vi "VPIExtraction.vi"() -> ()   [LabVIEW 2022 SP3]
uses:
  -planewaveSubs/VPIParams.ctl
  ViewData/-ReadEye/Header.ctl
  <vilib>/Utility/miscctls.llb/LVPointDoubleTypeDef.ctl
  <vilib>/Utility/error.llb/DialogType.ctl
  <vilib>/vision/Avi.llb/IMAQ AVI2 Codec Path.ctl
  ViewData/-ReadEye/TypeDefs/TypeofMean.ctl
  <vilib>/Analysis/baseanly.llb/Mean (DBL).vi
  <vilib>/Analysis/2dsp.llb/Decimate (single shot, DBL).vi
  <vilib>/Analysis/baseanly.llb/Normalize Matrix.vi
  <vilib>/Utility/file.llb/Write Delimited Spreadsheet (DBL).vi
  <vilib>/Utility/file.llb/Write Delimited Spreadsheet (string).vi
  <vilib>/Analysis/NI_AALBase.lvlib
  <vilib>/Analysis/NI_AALPro.lvlib
panel:
  in  "y scale Circ":sgl=1.0
  in  "Circle Mask":bool
  in  "RMS":bool
  in  "B1 Set":bool
  out "Header In":T1={"header info"={"Header"="", "Head length"=0}, "A/D info"={"# rf points per line"=0, "# lines per scan"=0, "sample rate MHz"=0, "# A/D bits"=0, "# bytes per A/D"=0, "TGC Flag"=0, "A/D Type"=""}, "Tranducer Info"={"bandwidth"=0.0, "center freq"=0.0, "start freq"=0.0, "ID"=0}, "Scan Info"={"delay"=0.0, "pivot distance"=0.0, "sector scan angle"=0.0, "operator"="", "Scan Mode"="", "location"=""}, "Time/Date Info"={"date"="", "time"=""}, "RF Info"={"RF file name"="", "RF file att"="", "RF cal file name"="", "RF cal file att"=""}, "Patient Info"={"ID"="", "extended ID"="", "age"=0, "sex"="", "previously\nscanned"="", "PSA"=0.0, "LOS"=1, "Ethnicty 2"=3, "Race"=3}, "Tissue Type"={"organ"=0, "disease type"=0, "disease location"=0, "IQ_pts"=0, "RcvBuffer"=0, "RcvFrame"=0, "IQBuff"=0, "IQFrame"=0, "IQPage"=0}, "Votage scaling"={"Digitizer (dB)"=0.0, "Gain (dB)"=0.0, "Atten (dB)"=0.0}, "Comment"="", "Misc Info"={"avg num"=0, "c speed"=0, "Div By or SF zones"=0, "XMIT CHS"=0, "RCV CHS"=0, "Xmit angle"=0.0}, "Therapy Parameters"={"Theraputic Freq (MHz)"=0.0, "Time on (s)"=0.0, "Therapy amplitude (mV)"=0.0, "Lines Before"=0, "Lines After"=0}, "Scan Settings"={"Energy (uJ or V)"=0, "Damp (Ohm) or Fc"=0, "HP Filt (KHz)"=0, "LP Filt (MHz)"=0, "Gain (db)"=0, "prf (kHz)"=0.0, "Distance between\nscan lines (um)"=0, "Distance between\nscan planes (um)"=0, "Scan line gap (um)"=0.0, "Scan plane gap (um)"=0.0}, "Compression Parameters"={"F1 (MHz)"=0.0, "F2 (MHz)"=0.0, "% taper"=0.0, "duration"=0.0}, "Patient Info Xtra"={"First Name"="", "Last Name"="", "Notes"=""}, "ROI Box"=[0, 0, 0, 0]} {"Compression Parameters"."% taper" min=50 max=1000 format="%.2f"; "Compression Parameters"."F2 (MHz)" format="%.3f"; "Compression Parameters"."F1 (MHz)" format="%.3f"; "Scan Settings"."prf (kHz)" format="%.2f"; "Therapy Parameters"."Therapy amplitude (mV)" min=50 max=1000 format="%.2f"; "Therapy Parameters"."Time on (s)" format="%.3f"; "Therapy Parameters"."Theraputic Freq (MHz)" format="%.3f"; "Patient Info"."Race" items=["Am Ind or Alaska", "Asian", "Hawaiian, Pac Isl", "Black or Afr Amer", "White", "more than one race", "unknown"]; "Patient Info"."Ethnicty 2" items=["Hispanic", "Non-Hispanic", "unknown"]; "Patient Info"."LOS" items=["1", "2", "3", "4", "5"]; "Patient Info"."PSA" format="%.1f"; "Scan Info"."delay" format="%.2f"; "Scan Info"."pivot distance" format="%.2f"; "Scan Info"."sector scan angle" format="%.2f"; "Tranducer Info"."bandwidth" format="%.2f"; "Tranducer Info"."center freq" format="%.2f"; "Tranducer Info"."start freq" format="%.2f"}
  in  "EKG Trace":path
  in  "No Mask?":bool=TRUE
  in  "Range Control":T2={"Vel Range"={1.4018691588785046, 50.0}, "PFlow Range"={22.429906542056074, 90.28037383177569}, "IQ Range"={28.037383177570092, 102.05607476635514}, "ShortLag"={33.08411214953271, 88.59813084112149}, "Mean Pow"={0.0, 41.12149532710281}, "powT"={0.0, 41.12149532710281}, "varT"={0.0, 41.12149532710281}} {"varT" scale=0.0..100.0; "powT" scale=0.0..700.0; "Mean Pow" scale=0.0..100.0; "ShortLag" scale=0.0..120.0; "IQ Range" scale=-25.0..120.0; "PFlow Range" scale=0.0..120.0; "Vel Range" scale=-1.0..150.0}
  in  "Main Tab":enum32{"Page 1", "Page 2", "Page 4"}(tab)=enum."Page 2"
  out "output cluster":T3
  out "powT":sgl[][](graph)
  out "VarT":sgl[][](graph)
  out "IQData (thresholdC=powerCMap)":sgl[][](graph)
  out "Mean varS":sgl[][](graph)
  out "powerFlow line":sgl[](graph)
  out "Short lag vs slow time VarS":sgl[](graph)
  out "Short lag variance VarS":sgl[][](graph)
  out "powerFlow (threshold = avg Var)":sgl[][](graph)
  out "Mean Pow":sgl[][](graph)
  out "Mean PowT":sgl[][](graph)
  out "Histogram Graph":T4(graph)
  in  "Max V":i32(slide)=24 scale=0.0..60.0
  in  "Save VPI JPGs":bool
  in  "Save Vels":bool
  out "Vel Y (cm/s) Main":sgl[][](graph)
  out "Velocity  vs time (cm/s)":dbl[][](graph)
  in  "AVG":i32=1 min=1
  in  "Operation":u16(ring) items=["Median", "Mean"]
  out "Vector Image":T5(plugin-control)
  out "SG":picture
  out "SG File":string
  out "Current  VPI":string
  in  "Card Cycles":i32=1
  out "CD Image":T5(plugin-control)
  in  "Location note":string
  in  "Skip":dbl=4.0
  in  "Skip overide?":bool
  out "Skip File":dbl
  in  "Tab Display":T6(tab)=enum."V at Marker"
  out "Vel Y (cm/s) Ref":sgl[][](graph)
  out "Vel mag (cm/s)":sgl[][](graph)
  out "Vel X (cm/s) Ref":sgl[][](graph)
  out "phase (cm/s)":sgl[][](graph)
  out "Raw Filtered":sgl[][](graph)
  in  "Frame":i32
  out "Velocity spread":cluster{"Y":dbl[], "Y":dbl[]}[](graph)
  out "Vel Sum (cm/s)":T7 {"Plane" min=0 step=1; "Curs Y" min=0 step=1; "Curs X" min=0 step=1}
  out "VelT":dbl[](graph)
  in  "length":i32=10
  in  "VPI Fix":cluster{"Offset":T8, "Scale":T8}={"Offset"={"X"=38.0, "Y"=10.0}, "Scale"={"X"=0.64, "Y"=0.82}}
  in  "CD Fix":cluster{"Offset":T8, "Scale":T8}={"Offset"={"X"=21.0, "Y"=19.0}, "Scale"={"X"=0.7, "Y"=0.673}}
  in  "SG Fix":cluster{"Start":dbl, "scale":dbl}={"Start"=55.0, "scale"=0.213}
  out "Velocity cut x-y plane (cm/s)":dbl[][](graph)
  out "Velocity cut  mean\nall time(cm/s)":dbl[][](graph)
  out "Flow Phase vs time":dbl[](graph)
  out "V mean running":dbl[][](array[numeric])
  out "V mean Var":dbl[][](array[numeric])
  out "Average vorticity vs time rot/s":dbl[][](graph)
  out "Energy loss vs time in window":dbl[](graph)
  in  "center zero":i32
  out "error%":dbl
  in  "rev/s":dbl=6.0
  out "mean vorticity":dbl format="%0.2f"
  out "Vorticity slow time":dbl[](graph)
  out "vorticy pixel\nmean across time":dbl format="%0.2f"
  in  "AVG #":i32=1 min=1
  in  "Vort Mean/Median":u16(ring) items=["Median", "Mean"]
  in  "vort frame  average":i32=3
  in  "step vort":i32=5
  in  "mean vort":bool
  in  "Save Vortex":bool
  out "KE vs time":dbl[](graph)
  in  "vort add char":string
  in  "downsamp factor":i32=10
  out "EKG":picture
  out "Peak Tracker":dbl[][](graph)
  in  "2D threshold":sgl=20.0
  in  "Ref Frame 2D CC":i32
  in  "#y rf":i32=80
  in  "#x lines":i32=100
  out "Simple Motion Tracker":dbl[](graph)
  out "Raw data (motion track marks)":sgl[][](graph)
  out "2D Correlation":dbl[][](graph)
  out "BPM":i32
  in  "True Center Freq":dbl=15.5
  in  "Save Images":bool
  in  "ImageSavePath":path=path "E:/Papers/IEEE/2109 VPI LV/FigsData"
  in  "VPI Case":i32 min=0
  out "Current":i32
  out "Total":i32
  out "Direction Map":picture
  in  "Direction cColor":picture
  in  "vort min val":dbl(slide) scale=0.0..1000.0
  out "z grid":cdb[][](array[numeric])
  in  "Values":T9
  in  "Plane":i32 min=0 step=1
  in  "stop":bool
  in  "Use Selected Files":bool
  in  "Listbox":i32[](listbox)
  in  "directory path of data and header file":path
  in  "search pattern":string="*VPI.raw"
  # "17.857 ref"
  # "Color based on net axial up or down"
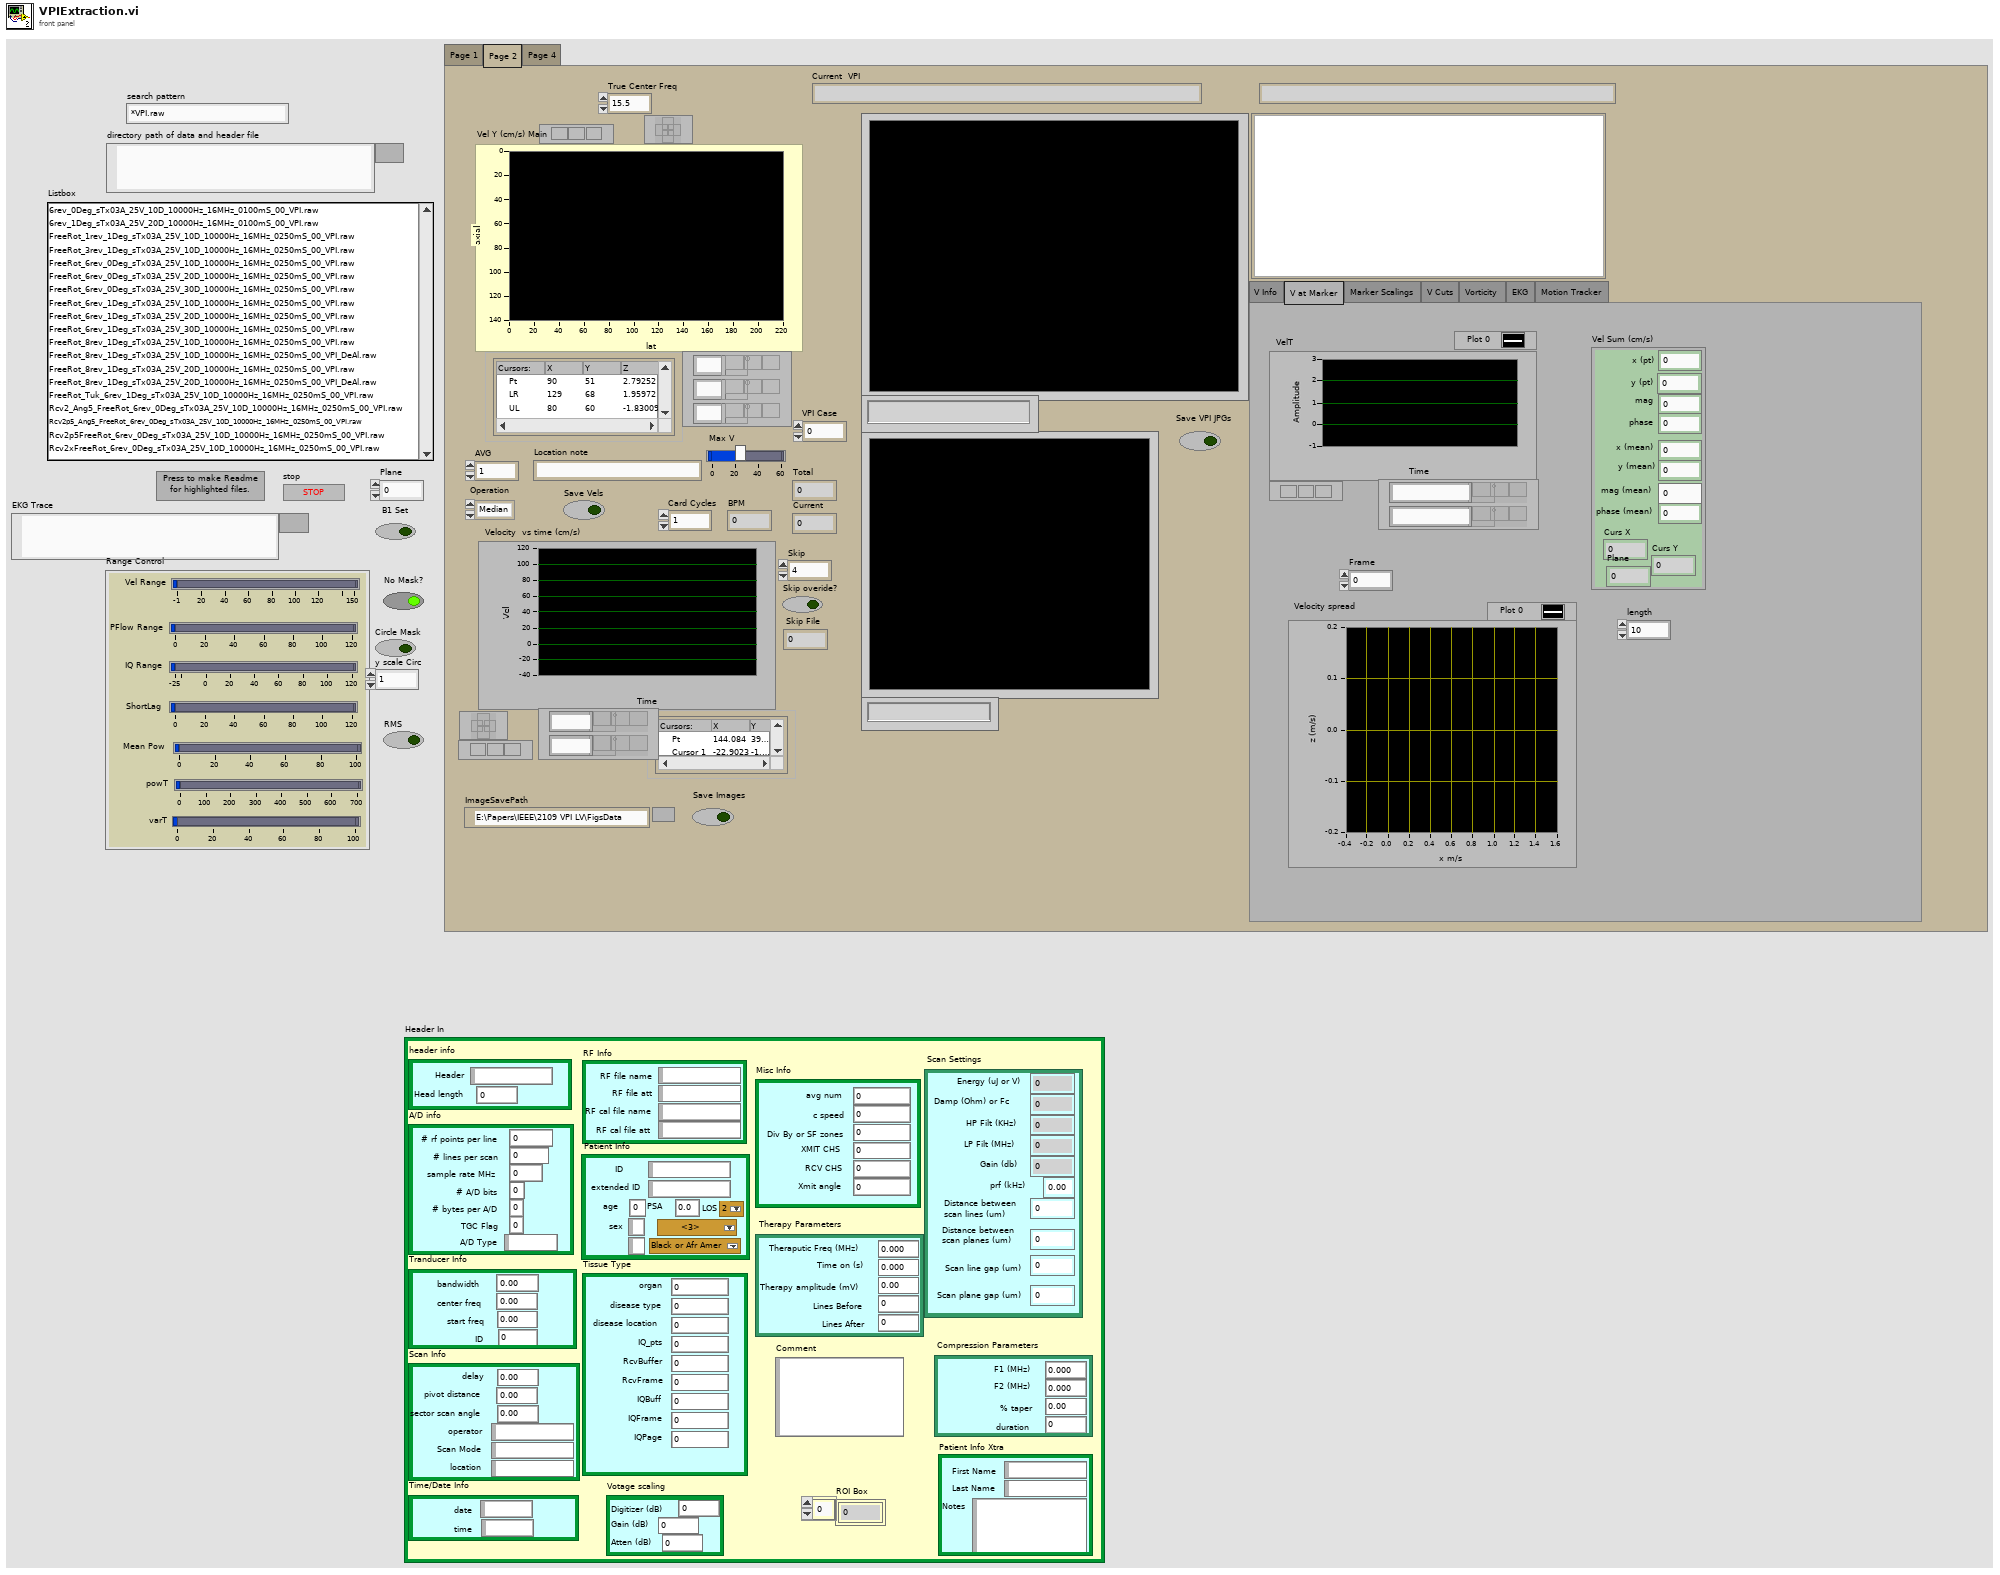
[diagram p1: front panel]
types:
  T1 = typedef "Header.ctl" = cluster{"header info":cluster{"Header":string, "Head length":i16}, "A/D info":cluster{"# rf points per line":u16, "# lines per scan":u16, "sample rate MHz":u16, "# A/D bits":i16, "# bytes per A/D":u16, "TGC Flag":u16, "A/D Type":string}, "Tranducer Info":cluster{"bandwidth":sgl, "center freq":sgl, "start freq":sgl, "ID":i32}, "Scan Info":cluster{"delay":sgl, "pivot distance":sgl, "sector scan angle":sgl, "operator":string, "Scan Mode":string, "location":string}, "Time/Date Info":cluster{"date":string, "time":string}, "RF Info":cluster{"RF file name":string, "RF file att":string, "RF cal file name":string, "RF cal file att":string}, "Patient Info":cluster{"ID":string, "extended ID":string, "age":u16, "sex":string, "previously\nscanned":string, "PSA":sgl, "LOS":u8, "Ethnicty 2":u8, "Race":u8}, "Tissue Type":cluster{"organ":i16, "disease type":i16, "disease location":i16, "IQ_pts":u16, "RcvBuffer":u8, "RcvFrame":u16, "IQBuff":u8, "IQFrame":u16, "IQPage":u8}, "Votage scaling":cluster{"Digitizer (dB)":sgl, "Gain (dB)":sgl, "Atten (dB)":sgl}, "Comment":string, "Misc Info":cluster{"avg num":u16, "c speed":i16, "Div By or SF zones":i16, "XMIT CHS":u8, "RCV CHS":u8, "Xmit angle":sgl}, "Therapy Parameters":cluster{"Theraputic Freq (MHz)":sgl, "Time on (s)":sgl, "Therapy amplitude (mV)":sgl, "Lines Before":u16, "Lines After":u16}, "Scan Settings":cluster{"Energy (uJ or V)":u8, "Damp (Ohm) or Fc":u8, "HP Filt (KHz)":u8, "LP Filt (MHz)":u8, "Gain (db)":u8, "prf (kHz)":sgl, "Distance between\nscan lines (um)":u16, "Distance between\nscan planes (um)":u16, "Scan line gap (um)":sgl, "Scan plane gap (um)":sgl}, "Compression Parameters":cluster{"F1 (MHz)":sgl, "F2 (MHz)":sgl, "% taper":sgl, "duration":sgl}, "Patient Info Xtra":cluster{"First Name":string, "Last Name":string, "Notes":string}, "ROI Box":u16[]}
  T2 = cluster{"Vel Range":cluster{dbl, dbl}, "PFlow Range":cluster{dbl, dbl}, "IQ Range":cluster{dbl, dbl}, "ShortLag":cluster{dbl, dbl}, "Mean Pow":cluster{dbl, dbl}, "powT":cluster{dbl, dbl}, "varT":cluster{dbl, dbl}}
  T3 = cluster{"Vel Max":sgl, "Vel Min":sgl, "PF Max":sgl, "PF Min":sgl, "IQ Max":sgl, "IQ Min":sgl, "ShortLag Max":sgl, "ShortLag Min":sgl, "MeanPow Max":sgl, "MeanPow Min":sgl, "powT max":sgl, "powT min":sgl, "varT max":sgl, "varT min":sgl}
  T4 = cluster{"X Values":dbl[], "Histogram: h(x)":i32[]}
  T5 = typedef "IMAQ Image.ctl" = refnum<image>
  T6 = enum32{"V Info", "V at Marker", "Marker Scalings", "V Cuts", "Vorticity", "EKG", "Motion Tracker"}
  T7 = cluster{"x (pt)":sgl, "y (pt)":sgl, "mag":sgl, "phase":sgl, "x (mean)":sgl, "y (mean)":sgl, "mag (mean)":sgl, "phase (mean)":sgl, "Curs X":sgl, "Curs Y":sgl, "Plane":sgl}
  T8 = typedef "LVPointDoubleTypeDef.ctl" = cluster{"X":dbl, "Y":dbl}
  T9 = typedef "VPIParams.ctl" = cluster{"xdim":dbl, "ydim":dbl, "zdim":dbl, "skip":dbl, "ensembleC":dbl, "ensembleVar\n":dbl, "#tx":dbl, "#Rx":dbl, "deltaX":dbl, "deltaY":dbl, "x start":dbl, "ystart":dbl}
  T10 = enum16{"big-endian, network order", "native, host order", "little-endian"}
  T11 = typedef "DialogType.ctl" = u16
  T12 = typedef "IMAQ AVI2 Codec Path.ctl" = u32
  T13 = typedef "IMAQ AVI2 Refnum.ctl" = refnum<k20>
  T14 = typedef "Image Type" = u32
  T15 = cluster{"AVI Refnum (duplicate)":T13, "New Image":T5, "appended path":path, sgl[][][], csg[][][], sgl[][][], "Values":T9, sgl[][][], "mean pow ":sgl[][], "mean var":sgl[][], "AVI Refnum (duplicate)":T13, "New Image":T5, "Number of Frames":u32, "Number of Frames":u32, sgl[][][], sgl[][][], sgl[][][], sgl[][][], "Header In":T1, "result string":string, sgl[][][]}
  T16 = typedef "TypeofMean.ctl" = enum16{"Mean from lines", "Mean just lines", "Poly Mean", "No mean", "Filter"}
  T17 = cluster{"abs(IQ)":sgl[][], "abs(IQ) SVD":sgl[][], "Vector out":csg[][], "pow":sgl[][], "vars short lag":sgl[][], "powT":sgl[][], "varT":sgl[][]}
  T18 = cluster{dbl, dbl, dbl, dbl, sgl, sgl, sgl, sgl, "Cursor X":dbl, "Cursor Y":dbl, "Plane":i32}
  T19 = typedef "NI_Matrix.lvlib/RealMatrix.ctl" = dbl[][]
  T20 = typedef "imagedata.ctl" = cluster{"image type":i32, "image depth":i32, "image":u8[], "mask":u8[], "colors":u32[], "Rectangle":cluster{"left":i16, "top":i16, "right":i16, "bottom":i16}}
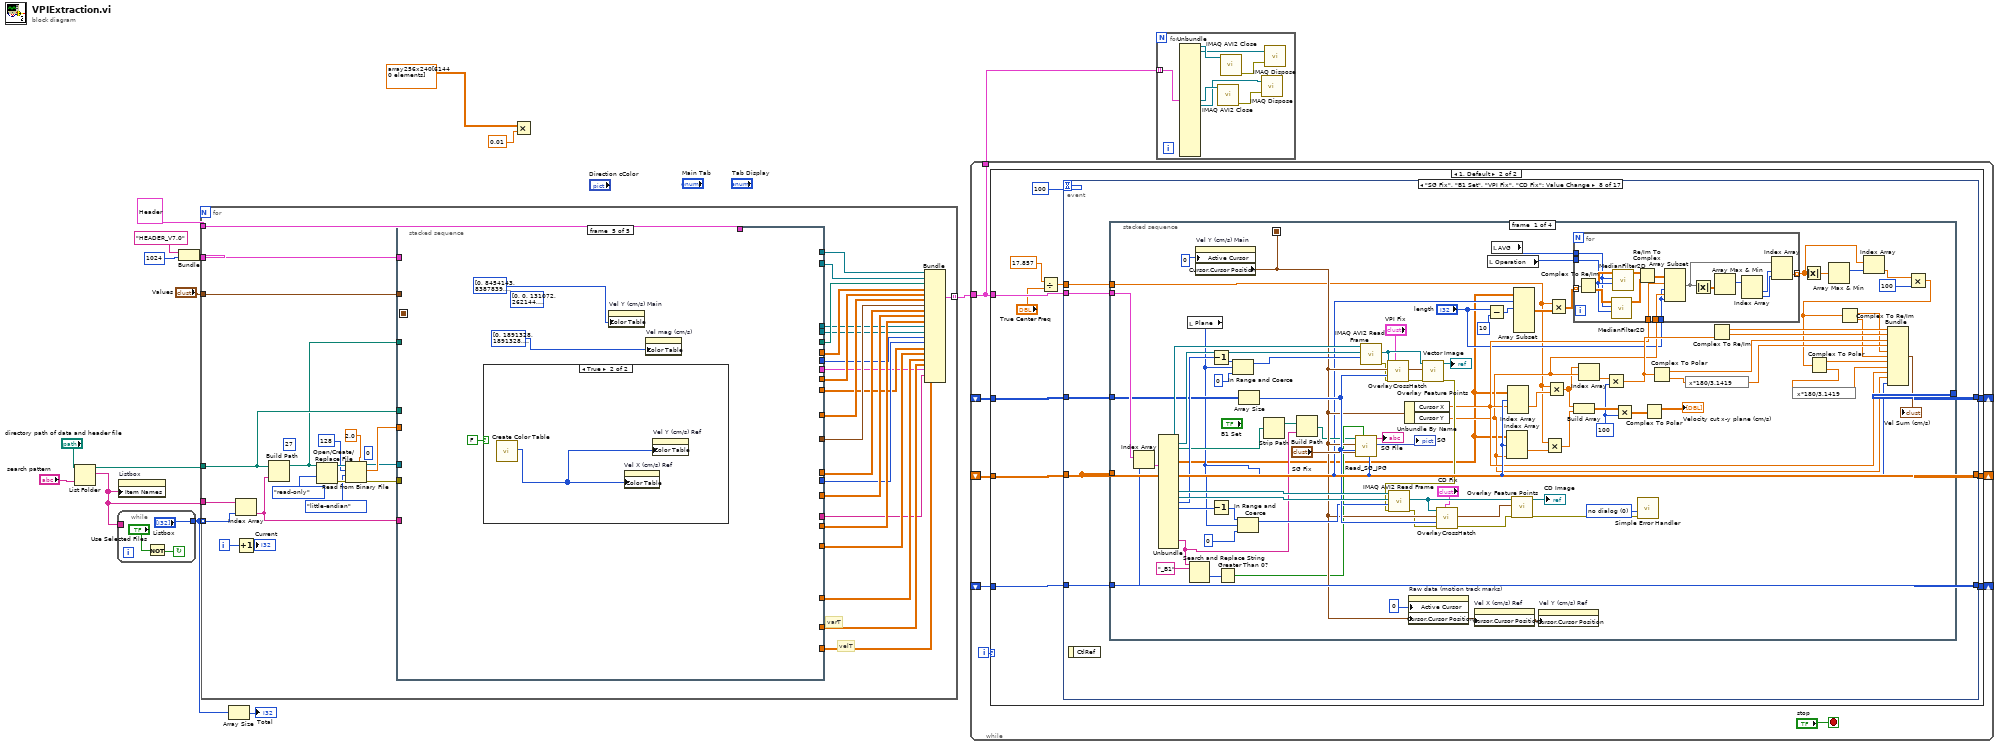
[diagram p0: block diagram]
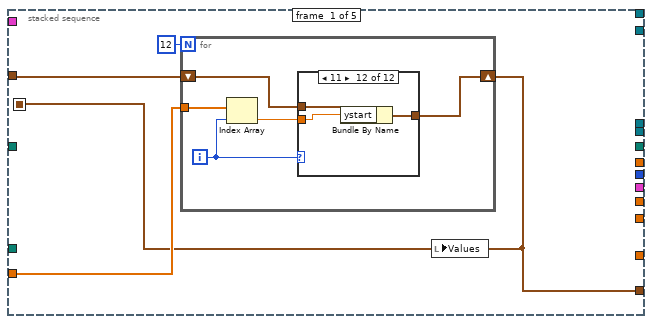
[diagram p2: hidden frame]
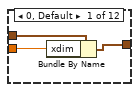
[diagram p3: hidden frame]
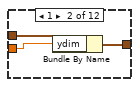
[diagram p4: hidden frame]
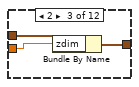
[diagram p5: hidden frame]
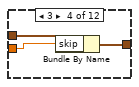
[diagram p6: hidden frame]
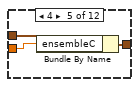
[diagram p7: hidden frame]
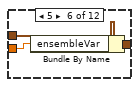
[diagram p8: hidden frame]
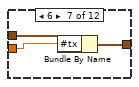
[diagram p9: hidden frame]
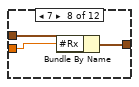
[diagram p10: hidden frame]
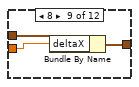
[diagram p11: hidden frame]
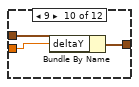
[diagram p12: hidden frame]
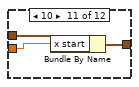
[diagram p13: hidden frame]
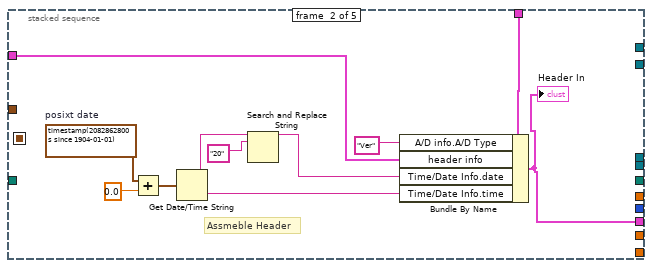
[diagram p14: hidden frame]
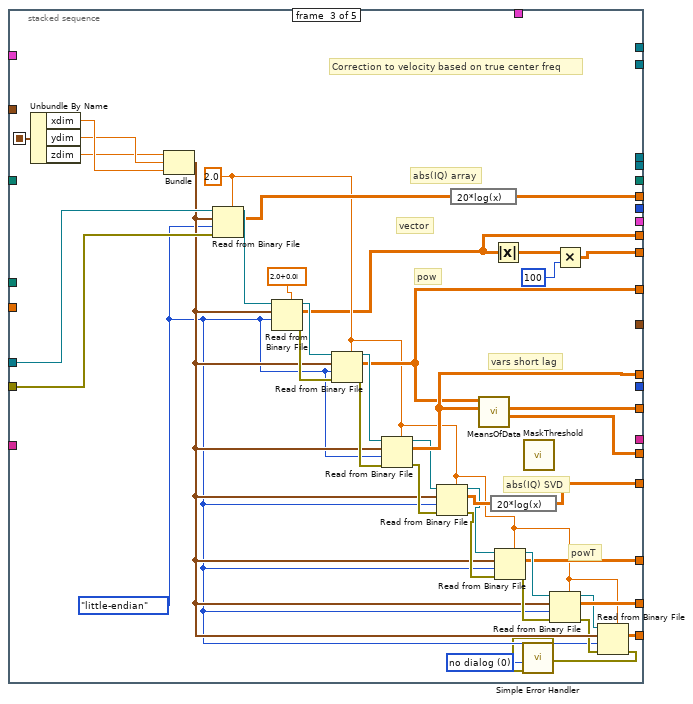
[diagram p15: hidden frame]
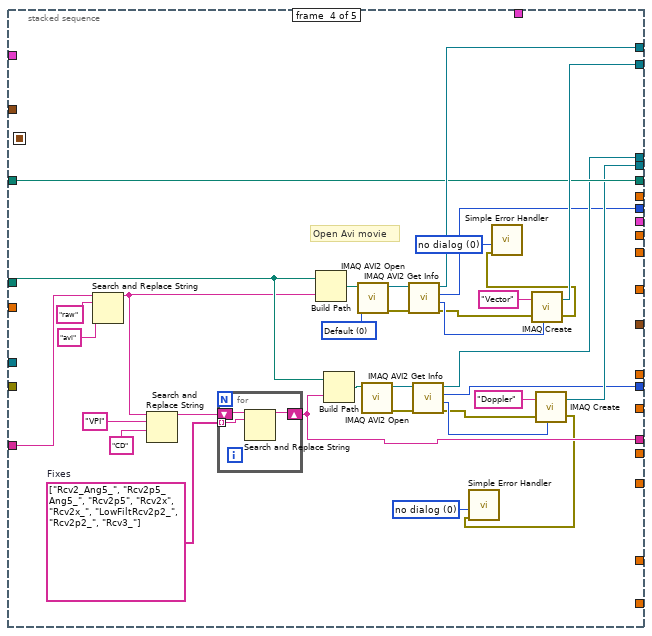
[diagram p16: hidden frame]
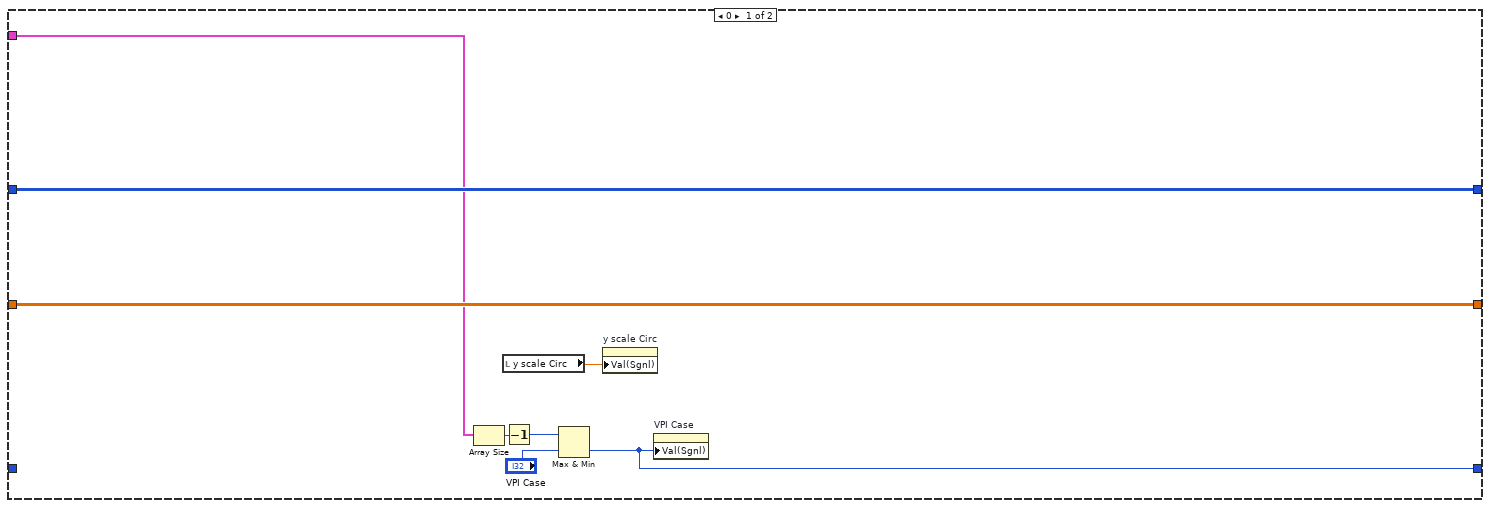
[diagram p18: hidden frame]
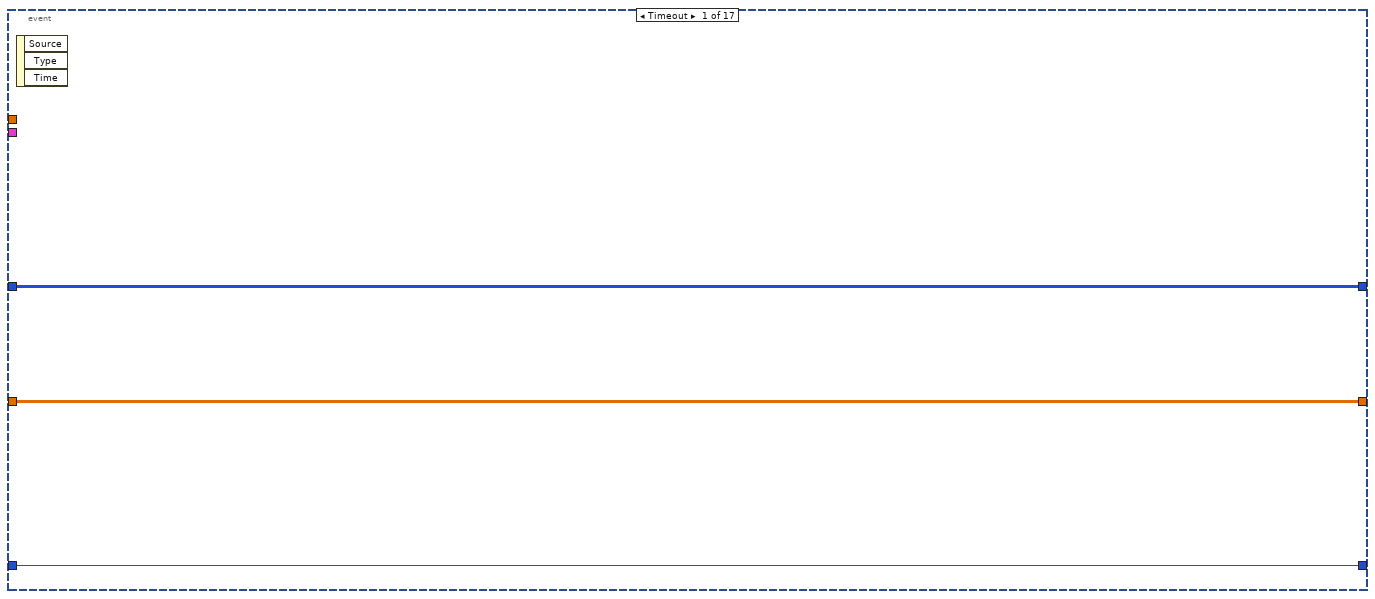
[diagram p19: hidden frame]
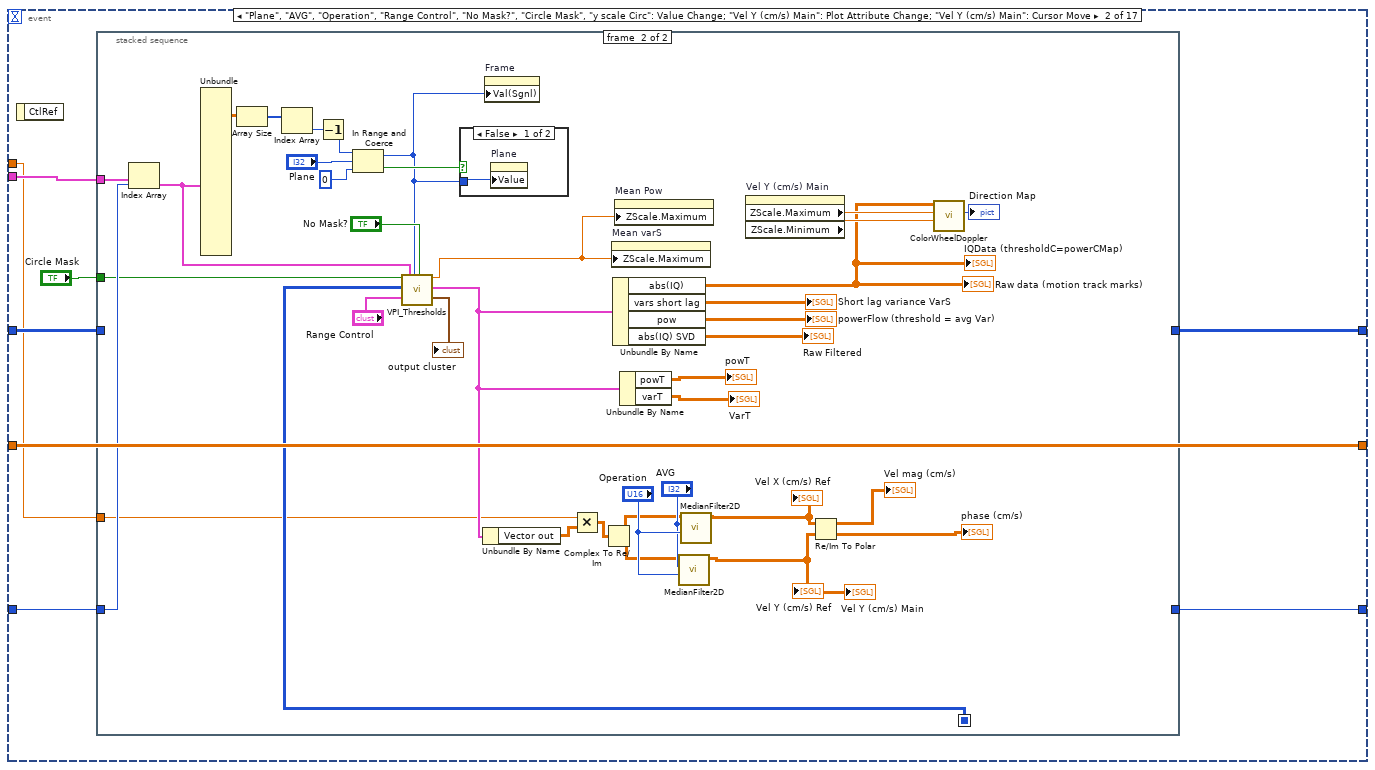
[diagram p20: hidden frame]
diagram:
  n1 = List Folder(path="directory path of data and header file", pattern="search pattern") -> (path out=w12:path, filenames=w11:string[])  [unwired: 1 in, 3 out]
  n2 = while {
    tunnel: ["Listbox"] -> w4
    tunnel: w11 -> [_]
    stop <- w18 continue-if-true
    n3 = Not(x="Use Selected Files") -> (.not. x?=w18:bool)
  }
  n4 = property on="Listbox" class="LstBox (strict)"("Item Names"=w11) -> ()  [unwired: 2 in, 2 out]
  n5 = Bundle("HEADER_V7.0", 1024) -> (w7:cluster{string, i32})  [unwired: 1 in]
  n6 = for {
    tunnel: w4 -> [w59] mode=indexing
    tunnel: w11 -> [w58]
    tunnel: w12 -> [w44]
    tunnel: T1 {"header info"={"Header"="", "Head length"=0}, "A/D info"={"# rf points per line"=0, "# lines per scan"=0, "sample rate MHz"=0, "# A/D bits"=0, "# bytes per A/D"=0, "TGC Flag"=0, "A/D Type"=""}, "Tranducer Info"={"bandwidth"=0.0, "center freq"=0.0, "start freq"=0.0, "ID"=0}, "Scan Info"={"delay"=0.0, "pivot distance"=0.0, "sector scan angle"=0.0, "operator"="", "Scan Mode"="", "location"=""}, "Time/Date Info"={"date"="", "time"=""}, "RF Info"={"RF file name"="", "RF file att"="", "RF cal file name"="", "RF cal file att"=""}, "Patient Info"={"ID"="", "extended ID"="", "age"=0, "sex"="", "previously\nscanned"="", "PSA"=0.0, "LOS"=1, "Ethnicty 2"=3, "Race"=3}, "Tissue Type"={"organ"=0, "disease type"=0, "disease location"=0, "IQ_pts"=0, "RcvBuffer"=0, "RcvFrame"=0, "IQBuff"=0, "IQFrame"=0, "IQPage"=0}, "Votage scaling"={"Digitizer (dB)"=0.0, "Gain (dB)"=0.0, "Atten (dB)"=0.0}, "Comment"="", "Misc Info"={"avg num"=0, "c speed"=0, "Div By or SF zones"=0, "XMIT CHS"=0, "RCV CHS"=0, "Xmit angle"=0.0}, "Therapy Parameters"={"Theraputic Freq (MHz)"=0.0, "Time on (s)"=0.0, "Therapy amplitude (mV)"=0.0, "Lines Before"=0, "Lines After"=0}, "Scan Settings"={"Energy (uJ or V)"=0, "Damp (Ohm) or Fc"=0, "HP Filt (KHz)"=0, "LP Filt (MHz)"=0, "Gain (db)"=0, "prf (kHz)"=0.0, "Distance between\nscan lines (um)"=0, "Distance between\nscan planes (um)"=0, "Scan line gap (um)"=0.0, "Scan plane gap (um)"=0.0}, "Compression Parameters"={"F1 (MHz)"=0.0, "F2 (MHz)"=0.0, "% taper"=0.0, "duration"=0.0}, "Patient Info Xtra"={"First Name"="", "Last Name"="", "Notes"=""}, "ROI Box"=[0, 0, 0, 0]} ("Header In") -> [w57]
    tunnel: w7 -> [w56]
    tunnel: "Values" -> [w49]
    tunnel: [w32] -> w15 mode=indexing
    i -> [w27]
    (unwired) u32 27 ("Column/Row to Sort By")
    (unwired) i64 0 ("offset (in bytes)")
    # "velT"
    # "varT"
    n7 = Index Array(array=w58, index=w59) -> (element=w45:string)
    n8 = Increment(x=w27) -> (x+1=→"Current":i32)
    n9 = Build Path(base path=w44, name or relative path=w45) -> (appended path=w43:path)
    n10 = Open/Create/Replace File(file path (use dialog)=w43, access (0:read/write)=enum16{"read/write", "read-only", "write-only"}."read-only") -> (refnum out=w54:refnum<file>, error out=w53:errorcluster)  [unwired: 4 in, 1 out]
    n11 = Read from Binary File(5:sgl 2.0 ("double"), 8:w53, 9:T10."little-endian" ("byte order (0:big-endian, network order)"), 10:128 ("count (1)"), 11:w54) -> (0:w47:errorcluster, 2:w50:sgl[], 3:w48:refnum<file>)  [unwired: 1 in, 1 out]
    n12 = stacked-sequence {
      seq-local: [w60 _ _ _ _] -> [_ _ w153 _ _]
      tunnel: w57 -> [_ w115 _ _ _]
      tunnel: w56 -> [_ w108 _ _ _]
      tunnel: w50 -> [w63 _ _ _ _]
      tunnel: w49 -> [w61 _ _ _ _]
      tunnel: w48 -> [_ _ w155 _ _]
      tunnel: w47 -> [_ _ w154 _ _]
      tunnel: [_ _ w143 _ _] -> w39
      tunnel: [_ _ w141 _ _] -> w37
      tunnel: [_ _ w116 _ _] -> w38
      tunnel: [_ _ w142 _ _] -> w35
      tunnel: [w60 _ _ _ _] -> w36
      tunnel: [_ _ w139 _ _] -> w33
      tunnel: [_ _ w140 _ _] -> w34
      tunnel: w45 -> [_ _ _ w165 _]
      tunnel: w44 -> [_ _ _ w172 _]
      tunnel: [_ _ _ w182 _] -> w41
      tunnel: [_ _ _ w181 _] -> w42
      tunnel: [_ _ _ w180 _] -> w40
      tunnel: w43 -> [_ _ _ w180 _]
      tunnel: [_ _ _ w170 _] -> w30
      tunnel: [_ _ _ w169 _] -> w31
      tunnel: [_ _ _ w168 _] -> w29
      tunnel: [_ _ _ w167 _] -> w28
      tunnel: [_ _ w136 _ _] -> w25
      tunnel: [_ _ w132 _ _] -> w24
      tunnel: [_ _ w127 _ _] -> w23
      tunnel: [_ _ w126 _ _] -> w22
      tunnel: [_ w105 _ _ _] -> w21
      tunnel: [_ _ _ w162 _] -> w20
      tunnel: [_ _ w119 _ _] -> w19
      frame #0 {
        n13 = for {
          N: 12 -> [_]
          tunnel: w63 -> [w68]
          shift-right: [w65] -> w60
          shift-left: w61 -> [w64]
          i -> [w66]
          n14 = Index Array(array=w68, index=w66) -> (element=w67:sgl)
          n15 = case shown="11" w66 {
            tunnel: w67 -> [w71 w74 w77 w80 w83 w86 w89 w92 w95 w98 w101 w104]
            tunnel: [w70 w73 w76 w79 w82 w85 w88 w91 w94 w97 w100 w103] -> w65
            tunnel: w64 -> [w69 w72 w75 w78 w81 w84 w87 w90 w93 w96 w99 w102]
            frame 0, Default {
              n16 = Bundle By Name(cluster=w69, "xdim"=w71) -> (w70:T9)
            }
            frame 1 {
              n17 = Bundle By Name(cluster=w72, "ydim"=w74) -> (w73:T9)
            }
            frame 2 {
              n18 = Bundle By Name(cluster=w75, "zdim"=w77) -> (w76:T9)
            }
            frame 3 {
              n19 = Bundle By Name(cluster=w78, "skip"=w80) -> (w79:T9)
            }
            frame 4 {
              n20 = Bundle By Name(cluster=w81, "ensembleC"=w83) -> (w82:T9)
            }
            frame 5 {
              n21 = Bundle By Name(cluster=w84, "ensembleVar"=w86) -> (w85:T9)
            }
            frame 6 {
              n22 = Bundle By Name(cluster=w87, "#tx"=w89) -> (w88:T9)
            }
            frame 7 {
              n23 = Bundle By Name(cluster=w90, "#Rx"=w92) -> (w91:T9)
            }
            frame 8 {
              n24 = Bundle By Name(cluster=w93, "deltaX"=w95) -> (w94:T9)
            }
            frame 9 {
              n25 = Bundle By Name(cluster=w96, "deltaY"=w98) -> (w97:T9)
            }
            frame 10 {
              n26 = Bundle By Name(cluster=w99, "x start"=w101) -> (w100:T9)
            }
            frame 11 {
              n27 = Bundle By Name(cluster=w102, "ystart"=w104) -> (w103:T9)
            }
          }
        }
        n28 = local write "Values"(w60) -> ()
      }
      frame #1 {
        w112 = timestamp(2082862800 s since 1904-01-01)  # posixt date
        # "Assmeble Header"
        n29 = Add(x=w112, y=0.0) -> (x+y=w114:timestamp)
        n30 = Get Date/Time String(seconds (now)=w114) -> (date string=w111:string, time string=w113:string)  [unwired: 2 in]
        n31 = Search and Replace String(input string=w111, search string="20") -> (result string=w109:string)  [unwired: 2 in, 7 out]
        n32 = Bundle By Name(cluster=w115, "A/D info.A/D Type"="Ver", "header info"=w108, "Time/Date Info.date"=w109, "Time/Date Info.time"=w113) -> (w105:T1)
        "Header In" <- w105
      }
      frame #2 {
        w117 = T11 0 items=["no dialog", "OK message", "continue or stop message", "OK message + warnings", "continue/stop + warnings"] ("type of dialog (OK msg:1)")
        w120 = T10."little-endian" ("byte order (0:big-endian, network order)")
        w123 = sgl 2.0 ("double")
        # "powT"
        # "Correction to velocity based on true center freq"
        # "abs(IQ) SVD"
        # "vars short lag"
        # "pow"
        # "vector"
        # "abs(IQ) array"
        n33 = Unbundle By Name(w153) -> ("xdim"=w152:dbl, "ydim"=w151:dbl, "zdim"=w125:dbl)
        n34 = Bundle("zdim"=w125, "ydim"=w151, "xdim"=w152) -> (w122:cluster{"zdim":dbl, "ydim":dbl, "xdim":dbl})  [unwired: 1 in]
        n35 = Read from Binary File(5:w123, 8:w154, 9:w120, 10:w122, 11:w155) -> (2:w144:sgl[][][], 3:w150:refnum<file>)  [unwired: 1 in, 2 out]
        n36 = Read from Binary File(5:csg 2.0+0.0i ("double"), 9:w120, 10:w122, 11:w150) -> (0:w147:errorcluster, 2:w116:csg[][][], 3:w145:refnum<file>)  [unwired: 2 in, 1 out]
        n37 = Read from Binary File(5:w123, 8:w147, 9:w120, 10:w122, 11:w145) -> (0:w146:errorcluster, 2:w141:sgl[][][], 3:w148:refnum<file>)  [unwired: 1 in, 1 out]
        n38 = Read from Binary File(5:w123, 8:w146, 9:w120, 10:w122, 11:w148) -> (0:w135:errorcluster, 2:w142:sgl[][][], 3:w134:refnum<file>)  [unwired: 1 in, 1 out]
        n39 = Read from Binary File(5:w123, 8:w135, 9:w120, 10:w122, 11:w134) -> (0:w130:errorcluster, 2:w133:sgl[][][], 3:w131:refnum<file>)  [unwired: 1 in, 1 out]
        n40 = expression code="20*log(x)"(w144) -> (w143:sgl[][][])
        n41 = call "MeansOfData.vi"("var"=w142, "pow"=w141) -> ("mean var"=w139:sgl[][], "mean pow"=w140:sgl[][])  [unwired: 7 in, 1 out]
        n42 = expression code="20*log(x)"(w133) -> (w132:sgl[][][])
        n43 = Absolute Value(x=w116) -> (abs(x)=w138:sgl[][][])
        n44 = Read from Binary File(5:w123, 8:w130, 9:w120, 10:w122, 11:w131) -> (0:w128:errorcluster, 2:w127:sgl[][][], 3:w129:refnum<file>)  [unwired: 1 in, 1 out]
        n45 = call "MaskThreshold.vi"() -> ()  [unwired: 11 in, 1 out]
        n46 = Read from Binary File(5:w123, 8:w128, 9:w120, 10:w122, 11:w129) -> (0:w121:errorcluster, 2:w126:sgl[][][], 3:w124:refnum<file>)  [unwired: 1 in, 1 out]
        n47 = Multiply(x=w138, y=100) -> (x*y=w136:sgl[][][])
        n48 = Read from Binary File(5:w123, 8:w121, 9:w120, 10:w122, 11:w124) -> (0:w118:errorcluster, 2:w119:sgl[][][])  [unwired: 1 in, 2 out]
        n49 = call <vilib>:"Simple Error Handler.vi"("type of dialog (OK msg:1)"=w117, "error in (no error)"=w118) -> ()  [unwired: 3 in, 5 out]
      }
      frame #3 {
        w159 = T11 0 items=["no dialog", "OK message", "continue or stop message", "OK message + warnings", "continue/stop + warnings"] ("type of dialog (OK msg:1)")
        w161 = T11 0 items=["no dialog", "OK message", "continue or stop message", "OK message + warnings", "continue/stop + warnings"] ("type of dialog (OK msg:1)")
        w163 = string[] ["Rcv2_Ang5_", "Rcv2p5_Ang5_", "Rcv2p5", "Rcv2x", "Rcv2x_", "LowFiltRcv2p2_", "Rcv2p2_", "Rcv3_"]  # Fixes
        w166 = T12 0 items=["Default", "System", "Built in Vision"] ("Codec Source")
        # "Open Avi movie"
        n50 = Search and Replace String(input string=w165, search string="raw", replace string="avi" ("replace string (\"\")")) -> (result string=w171:string)  [unwired: 5 in, 3 out]
        n51 = Search and Replace String(input string=w171, search string="VPI", replace string="CD" ("replace string (\"\")")) -> (result string=w164:string)  [unwired: 5 in, 3 out]
        n52 = for {
          tunnel: w163 -> [w191] mode=indexing
          shift-right: [w190] -> w162
          shift-left: w164 -> [w192]
          n53 = Search and Replace String(input string=w192, search string=w191) -> (result string=w190:string)  [unwired: 6 in, 3 out]
        }
        n54 = Build Path(base path=w172, name or relative path=w171) -> (appended path=w183:path)
        n55 = Build Path(base path=w172, name or relative path=w162) -> (appended path=w173:path)
        n56 = call "IMAQ AVI2 Open"("Codec Source"=w166, "AVI File Path"=w183) -> ("error out"=w188:errorcluster, "AVI Refnum"=w187:T13)  [unwired: 1 in, 7 out]
        n57 = call "IMAQ AVI2 Open"("AVI File Path"=w173) -> ("error out"=w178:errorcluster, "AVI Refnum"=w177:T13)  [unwired: 2 in, 7 out]
        n58 = call "IMAQ AVI2 Get Info"("error in (no error)"=w188, "AVI Refnum"=w187) -> ("error out"=w158:errorcluster, "Image Type"=w186:T14, "Number of Frames"=w168:u32, "AVI Refnum (duplicate)"=w181:T13)  [unwired: 6 out]
        n59 = call "IMAQ AVI2 Get Info"("error in (no error)"=w178, "AVI Refnum"=w177) -> ("error out"=w160:errorcluster, "Image Type"=w176:T14, "Number of Frames"=w167:u32, "AVI Refnum (duplicate)"=w169:T13)  [unwired: 6 out]
        n60 = call "IMAQ Create"("Image Name"="Vector", "Image Type"=w186, "error in (no error)"=w158) -> ("New Image"=w182:T5, "error out"=w156:errorcluster)  [unwired: 1 in, 1 out]
        n61 = call <vilib>:"Simple Error Handler.vi"("type of dialog (OK msg:1)"=w159, "error in (no error)"=w156) -> ()  [unwired: 3 in, 5 out]
        n62 = call "IMAQ Create"("Image Name"="Doppler", "Image Type"=w176, "error in (no error)"=w160) -> ("New Image"=w170:T5, "error out"=w157:errorcluster)  [unwired: 1 in, 1 out]
        n63 = call <vilib>:"Simple Error Handler.vi"("type of dialog (OK msg:1)"=w161, "error in (no error)"=w157) -> ()  [unwired: 3 in, 5 out]
      }
      frame #4 {
        (unwired) u32[] [0, 0, 131072, 262144, 393216, 524288, 655360, 786432, 917504, 1048576, 1179648, 1310720, 1441792, 1572864, 1703936, 1835008, 1966080, 2097152, 2228224, 2359296, 2490368, 2621440, 2752512, 2883584, 3014656, 3145728, 3276800, 3407872, 3538944, 3670016, 3801088, 3932160, 4063232, 4194304, 4325376, 4456448, 4587520, 4718592, 4849664, 4980736, 5111808, 5242880, 5373952, 5505024, 5636096, 5767168, 5898240, 6029312, 6160384, 6291456, 6422528, 6553600, 6684672, 6815744, 6946816, 7077888, 7208960, 7340032, 7471104, 7602176, 7733248, 7864320, 7995392, 8126464, 8257536, 8388608, 8519680, 8650752, 8781824, 8912896, 9043968, 9175040, 9306112, 9437184, 9568256, 9699328, 9830400, 9961472, 10092544, 10223616, 10354688, 10485760, 10616832, 10747904, 10878976, 11010048, 11141120, 11272192, 11403264, 11534336, 11665408, 11796480, 11927552, 12058624, 12189696, 12320768, 12451840, 12582912, 12713984, 12845056, 12976128, 13107200, 13238272, 13369344, 13500416, 13631488, 13762560, 13893632, 14024704, 14155776, 14286848, 14417920, 14548992, 14680064, 14811136, 14942208, 15073280, 15204352, 15335424, 15466496, 15597568, 15728640, 15859712, 15990784, 16121856, 16252928, 16384000, 16515072, 16646144, 16712192, 16712704, 16713216, 16713728, 16714240, 16714752, 16715264, 16715776, 16716288, 16716800, 16717312, 16717824, 16718336, 16718848, 16719360, 16719872, 16720384, 16720896, 16721408, 16721920, 16722432, 16722944, 16723456, 16723968, 16724480, 16724992, 16725504, 16726016, 16726528, 16727040, 16727552, 16728064, 16728576, 16729088, 16729600, 16730112, 16730624, 16731136, 16731648, 16732160, 16732672, 16733184, 16733696, 16734208, 16734720, 16735232, 16735744, 16736256, 16736768, 16737280, 16737792, 16738304, 16738816, 16739328, 16739840, 16740352, 16740864, 16741376, 16741888, 16742400, 16742912, 16743424, 16743936, 16744448, 16744960, 16745472, 16745984, 16746496, 16747008, 16747520, 16748032, 16748544, 16749056, 16749568, 16750080, 16750592, 16751104, 16751616, 16752128, 16752640, 16753152, 16753664, 16754176, 16754688, 16755200, 16755712, 16756224, 16756736, 16757248, 16757760, 16758272, 16758784, 16759296, 16759808, 16760320, 16760832, 16761344, 16761856, 16762368, 16762880, 16763392, 16763904, 16764416, 16764928, 16765440, 16765952, 16766464, 16766976, 16767488, 16768000, 16768512, 16769024, 16769536, 16770048, 16770560, 16771072, 16771584, 16772096, 16772608, 16773120, 16773632, 16774144, 16774656, 16775168, 16775680, 16776192, 16777215] ("Color Table")
        n64 = case shown="True" FALSE {
          frame False {
          }
          frame True {
            n65 = call "Create Color Table.vi"() -> ("Color Table"=w196:u32[])  [unwired: 10 in, 1 out]
            n66 = property on="Vel X (cm/s) Ref" class="IntGraph (strict)"("Color Table"=w196) -> ()  [unwired: 2 in, 2 out]
            n67 = property on="Vel Y (cm/s) Ref" class="IntGraph (strict)"("Color Table"=w196) -> ()  [unwired: 2 in, 2 out]
          }
        }
        n68 = property on="Vel Y (cm/s) Main" class="IntGraph (strict)"("Color Table"=u32[] [0, 8454143, 8387839, 8255743, 8189183, 8057343, 7990783, 7858687, 7792127, 7660287, 7593727, 7461631, 7395071, 7263231, 7131135, 7064575, 6932735, 6866175, 6734079, 6667519, 6535679, 6469119, 6337023, 6270463, 6138623, 6006527, 5939967, 5807871, 5741567, 5609471, 5542911, 5411071, 5344511, 5212415, 5145855, 5014015, 4881919, 4815359, 4683263, 4616959, 4484863, 4418303, 4286207, 4219903, 4087807, 4021247, 3889407, 3822847, 3690751, 3558655, 3492351, 3360255, 3293695, 3161599, 3095295, 2963199, 2896639, 2764543, 2698239, 2566143, 2434047, 2367743, 2235647, 2169087, 2036991, 1970940, 1970936, 1905396, 1905392, 1839596, 1839592, 1774052, 1773792, 1708252, 1708248, 1708244, 1642448, 1642444, 1576904, 1576644, 1511104, 1511100, 1445560, 1445300, 1379760, 1379756, 1313960, 1313956, 1248416, 1248412, 1182616, 1182612, 1182608, 1116812, 1116808, 1051268, 1051264, 985468, 985464, 919924, 919664, 854124, 854120, 788580, 788320, 722780, 722776, 656980, 656976, 591436, 591432, 591172, 525632, 525628, 459832, 459828, 394288, 394284, 328488, 328484, 262944, 262684, 197144, 197140, 131600, 131340, 65800, 65796, 65792, 262144, 524288, 786432, 1048576, 1310720, 1572864, 1835008, 2097152, 2359296, 2621440, 2883584, 3145728, 3407872, 3670016, 3932160, 4194304, 4456448, 4718592, 4980736, 5242880, 5505024, 5767168, 6029312, 6291456, 6553600, 6815744, 7077888, 7340032, 7602176, 7864320, 8126464, 8388608, 8650752, 8912896, 9175040, 9437184, 9699328, 9961472, 10223616, 10485760, 10747904, 11010048, 11272192, 11534336, 11796480, 12058624, 12320768, 12582912, 12845056, 13107200, 13369344, 13631488, 13893632, 14155776, 14417920, 14680064, 14942208, 15204352, 15466496, 15728640, 15990784, 16252928, 16515072, 16712192, 16713216, 16714240, 16715264, 16716288, 16717312, 16718336, 16719360, 16720384, 16721408, 16722432, 16723456, 16724480, 16725504, 16726528, 16727552, 16728576, 16729600, 16730624, 16731648, 16732672, 16733696, 16734720, 16735744, 16736768, 16737792, 16738816, 16739840, 16740864, 16741888, 16742912, 16743936, 16744960, 16745984, 16747008, 16748032, 16749056, 16750080, 16751104, 16752128, 16753152, 16754176, 16755200, 16756224, 16757248, 16758272, 16759296, 16760320, 16761344, 16762368, 16763392, 16764416, 16765440, 16766464, 16767488, 16768512, 16769536, 16770560, 16771584, 16772608, 16773632, 16774656, 16775680, 16777215]) -> ()  [unwired: 2 in, 2 out]
        n69 = property on="Vel mag (cm/s)" class="IntGraph (strict)"("Color Table"=u32[] [0, 1891328, 1891328, 1891584, 1957120, 1957376, 1957376, 2023168, 2023168, 2088960, 2088960, 2089216, 2155008, 2155008, 2220800, 2220800, 2221056, 2286592, 2286848, 2352384, 2352640, 2352896, 2418432, 2418688, 2484224, 2484480, 2484480, 2550272, 2550272, 2616064, 2616064, 2616320, 2682112, 2682112, 2682368, 2747904, 2748160, 2813696, 2813952, 2813952, 2879744, 2880000, 2945536, 2945792, 2945792, 3011584, 3011584, 3077376, 3077376, 3077632, 3143424, 3143424, 3209216, 3209216, 3209472, 3275008, 3275264, 3340800, 3341056, 3341056, 3406848, 3407104, 3472640, 3472896, 3472896, 3604224, 3800832, 3997184, 4259072, 4455680, 4652032, 4848384, 5044992, 5306880, 5503232, 5699840, 5896192, 6092544, 6289152, 6551040, 6747392, 6944000, 7140352, 7336704, 7598848, 7795200, 7991552, 8188160, 8384512, 8580864, 8843008, 9039360, 9235712, 9432320, 9628672, 9890560, 10087168, 10283520, 10479872, 10676480, 10872832, 11134720, 11331328, 11527680, 11724032, 11920640, 12182528, 12378880, 12575488, 12771840, 12968192, 13164800, 13426688, 13623040, 13819648, 14016000, 14212352, 14474496, 14670848, 14867200, 15063808, 15260160, 15456512, 15718656, 15915008, 16111360, 16307968, 16504320, 16700928, 16765952, 16765440, 16765184, 16764673, 16764417, 16763905, 16763649, 16763138, 16762626, 16762370, 16761859, 16761603, 16761091, 16760835, 16760324, 16760068, 16759556, 16759045, 16758789, 16758277, 16758021, 16757510, 16757254, 16756742, 16756487, 16755975, 16755463, 16755207, 16754696, 16754440, 16753928, 16753673, 16753161, 16752649, 16752393, 16751882, 16751626, 16751114, 16750859, 16750347, 16750091, 16749579, 16749068, 16748812, 16748300, 16748045, 16747533, 16747277, 16746765, 16746510, 16745998, 16745486, 16745231, 16744719, 16744463, 16743951, 16743696, 16743184, 16742928, 16742417, 16741905, 16741649, 16741137, 16740881, 16740369, 16739857, 16739345, 16738832, 16738576, 16738064, 16737551, 16737039, 16736527, 16736271, 16735758, 16735246, 16734734, 16734221, 16733965, 16733453, 16732941, 16732428, 16731916, 16731660, 16731147, 16730635, 16730123, 16729867, 16729354, 16728842, 16728330, 16727817, 16727561, 16727049, 16726537, 16726024, 16725512, 16725256, 16724743, 16724231, 16723719, 16723207, 16722950, 16722438, 16721926, 16721413, 16720901, 16720645, 16720133, 16719620, 16719108, 16718596, 16718339, 16717827, 16717315, 16716803, 16716290, 16716034, 16715522, 16715009, 16714497, 16713985, 16713729, 16713216, 16712704, 16712192, 16777215]) -> ()  [unwired: 2 in, 2 out]
      }
    }
    n70 = Bundle("AVI Refnum (duplicate)"=w42, "New Image"=w41, "appended path"=w40, w39, w38, w37, "Values"=w36, w35, "mean pow"=w34, "mean var"=w33, "AVI Refnum (duplicate)"=w31, "New Image"=w30, "Number of Frames"=w29, "Number of Frames"=w28, w25, w24, w23, w22, "Header In"=w21, "result string"=w20, w19) -> (w32:T15)  [unwired: 1 in]
  }
  n71 = Array Size(array=w4) -> (size(s)=→"Total":i32)
  n72 = Multiply(x=cdb[][] array256x240[61440 elements] ("result"), y=0.01) -> ()  [unwired: 1 out]
  n73 = while {
    shift-right: [w204] -> _
    shift-left: _ -> [w203]
    shift-right: [w202] -> _
    shift-left: _ -> [w201]
    tunnel: w15 -> [w200]
    tunnel: [w200] -> w14
    shift-right: [w199] -> _
    shift-left: _ -> [w198]
    i -> [w197]
    stop <- "stop" stop-if-true
    n74 = case shown="1, Default" w197 {
      tunnel: [w213 w217] -> w204
      tunnel: w203 -> [w213 w218]
      tunnel: [w212 w224] -> w202
      tunnel: w201 -> [w212 w223]
      tunnel: w200 -> [w210 w222]
      tunnel: [w207 w220] -> w199
      tunnel: w198 -> [_ w219]
      frame 0 {
        n75 = Array Size(array=w210) -> (size(s)=w209:i32)
        n76 = local read "y scale Circ"() -> (w211:sgl)
        n77 = Decrement(x=w209) -> (x-1=w206:i32)
        n78 = Max & Min(x=w206, y="VPI Case") -> (min(x,y)=w207:i32)  [unwired: 1 out]
        n79 = property on="y scale Circ" class="DigNum (strict)"("Val(Sgnl)"=w211) -> ()  [unwired: 2 in, 2 out]
        n80 = property on="VPI Case" class="DigNum (strict)"("Val(Sgnl)"=w207) -> ()  [unwired: 2 in, 2 out]
      }
      frame 1, Default {
        n81 = Divide(x=17.857, y="True Center Freq") -> (x/y=w214:dbl)
        n82 = event shown="[7] \"SG Fix\", \"B1 Set\", \"VPI Fix\", \"CD Fix\": Value Change" {
          selector: _ -> [_ _ _ _ _ _ _ _ _ _ _ _ _ _ _ _ _]
          dyn-events: _ -> [_ _ _ _ _ _ _ _ _ _ _ _ _ _ _ _ _]
          timeout: 100 -> [_ _ _ _ _ _ _ _ _ _ _ _ _ _ _ _ _]
          tunnel: [w227 w235 w306 w325 w357 w390 w412 w451 w656 w673 w700 w735 w753 w788 w799 w851 w857] -> w224
          tunnel: w223 -> [w227 w235 w306 w325 _ w390 w412 w451 w656 w673 w700 w735 w753 w788 w799 w851 w857]
          tunnel: [_ _ _ _ _ _ _ w451 _ w673 _ _ _ _ _ _ _] -> _
          tunnel: w222 -> [_ w234 w302 w323 w355 w376 w431 w453 _ w675 w696 w734 w752 w785 _ w848 _]
          tunnel: [w226 w230 w301 w321 w352 w377 w411 w452 w655 w674 w698 w733 w748 w782 w798 w850 w856] -> w220
          tunnel: w219 -> [w226 w233 w301 w321 w352 w377 w411 w452 w655 w674 w698 w733 w748 _ w798 w850 w856]
          tunnel: w218 -> [w225 w229 w299 w308 w334 w389 w419 w450 w654 w670 w683 w708 w747 w768 w794 w849 w855]
          tunnel: [w225 w232 w299 w308 w334 w389 w419 w449 w654 w670 w683 w708 w747 w768 w794 w849 w855] -> w217
          tunnel: w214 -> [_ w228 w298 _ w331 w363 _ w448 _ _ _ _ _ _ _ _ _]
          event Timeout {
            n83 = event-data() -> ()  [unwired: 1 in, 3 out]
          }
          event "Plane", "AVG", "Operation", "Range Control", "No Mask?", "Circle Mask", "y scale Circ": Value Change; "Vel Y (cm/s) Main": Plot Attribute Change; "Vel Y (cm/s) Main": Cursor Move {
            n84 = event-data() -> ()  [unwired: 1 in, 1 out]
            n85 = stacked-sequence {
              seq-local: [w240 _] -> [_ w270]
              tunnel: w234 -> [w241 w283]
              tunnel: w233 -> [w237 w281]
              tunnel: [w240 _] -> w232
              tunnel: "Circle Mask" -> [w238 w269]
              tunnel: [w237 _] -> w230
              tunnel: w229 -> [_ _]
              tunnel: w228 -> [_ w258]
              frame #0 {
                n86 = Index Array(array=w241, index=w237) -> (element=w242:T15)
                n87 = local read "B1 Set"() -> (w236:bool)
                n88 = Unbundle(w242) -> (w239:sgl[][][])  [unwired: 20 out]
                n89 = property on="B1 Set" class="Bool (strict)"("Val(Sgnl)"=w236) -> ()  [unwired: 2 in, 2 out]
                n90 = case shown="True" w238 {
                  tunnel: [w244 w256] -> w240
                  tunnel: w239 -> [w243 w250]
                  frame False {
                    n91 = Index Array(array=w243, index (dim 0)=0 ("index (page)")) -> (element=w246:sgl[][])  [unwired: 2 in]
                    n92 = expression code="x*0+1"(w246) -> (w247:sgl[][])
                    n93 = To Word Integer(number=w247) -> (16bit integer=w244:i16[][])
                  }
                  frame True {
                    n94 = property on="Vel Y (cm/s) Main" class="IntGraph (strict)"("Active Cursor"=u32 1, "Active Cursor"=u32 2) -> ("Cursor.Cursor Position"=w255:T8, "Cursor.Cursor Position"=w251:T8)  [unwired: 2 in, 2 out]
                    n95 = Index Array(array=w250) -> (element=w249:sgl[][])  [unwired: 3 in]
                    n96 = call "CircleMask.vi"("y scale"="y scale Circ", "Array in"=w249, "Cursor 1"=w251, "Cursor 0"=w255) -> ("Array 3"=w256:i16[][], "Coordinates"=→"z grid":cdb[][])  [unwired: 6 in]
                  }
                }
              }
              frame #1 {
                n97 = Index Array(array=w283, index=w281) -> (element=w279:T15)
                n98 = Unbundle(w279) -> (w282:sgl[][][])  [unwired: 20 out]
                n99 = Array Size(array=w282) -> (size(s)=w286:i32[])
                n100 = Index Array(array=w286) -> (element=w285:i32)  [unwired: 1 in]
                n101 = Decrement(x=w285) -> (x-1=w280:i32)
                n102 = In Range and Coerce(upper limit=w280, x="Plane", lower limit=0) -> (coerced(x)=w260:i32, In Range?=w284:bool)
                n103 = call "VPI_Thresholds.vi"("Circle Mask"=w269, "mask"=w270, "GThresholds"="Range Control", "Datea items"=w279, "Plane"=w260, "No Mask?"="No Mask?") -> ("Max MeanVarS"=w291:dbl, "Outputs"=w271:T17, "output cluster"=→"output cluster":T3)  [unwired: 10 in, 1 out]
                n104 = case shown="False" w284 {
                  tunnel: w260 -> [w295 _]
                  frame False {
                    n105 = property on="Plane" class="DigNum (strict)"("Value"=w295) -> ()  [unwired: 2 in, 2 out]
                  }
                  frame True {
                  }
                }
                n106 = Unbundle By Name(w271) -> ("Vector out"=w259:csg[][])
                n107 = property on="Frame" class="DigNum (strict)"("Val(Sgnl)"=w260) -> ()  [unwired: 2 in, 2 out]
                n108 = Multiply(x=w258, y=w259) -> (x*y=w257:cdb[][])
                n109 = Complex To Re/Im(x + iy=w257) -> (x=w266:dbl[][], y=w265:dbl[][])
                n110 = property on="Mean varS" class="IntGraph (strict)"("ZScale.Maximum"=w291) -> ()  [unwired: 2 in, 2 out]
                n111 = Unbundle By Name(w271) -> ("abs(IQ)"=w278:sgl[][], "vars short lag"=→"Short lag variance VarS":sgl[][], "pow"=→"powerFlow (threshold = avg Var)":sgl[][], "abs(IQ) SVD"=→"Raw Filtered":sgl[][])
                "Raw data (motion track marks)" <- w278
                "IQData (thresholdC=powerCMap)" <- w278
                n112 = property on="Mean Pow" class="IntGraph (strict)"("ZScale.Maximum"=w291) -> ()  [unwired: 2 in, 2 out]
                n113 = Unbundle By Name(w271) -> ("powT"=→"powT":sgl[][], "varT"=→"VarT":sgl[][])
                n114 = call "MedianFilter2D.vi"("Operation"="Operation", "Pts to use"="AVG", "Raw In"=w265) -> ("output array"=w263:sgl[][])  [unwired: 8 in]
                "Vel Y (cm/s) Ref" <- w263
                "Vel Y (cm/s) Main" <- w263
                n115 = call "MedianFilter2D.vi"("Operation"="Operation", "Pts to use"="AVG", "Raw In"=w266) -> ("output array"=w264:sgl[][])  [unwired: 8 in]
                "Vel X (cm/s) Ref" <- w264
                n116 = property on="Vel Y (cm/s) Main" class="IntGraph (strict)"() -> ("ZScale.Maximum"=w294:dbl, "ZScale.Minimum"=w292:dbl)  [unwired: 2 in, 2 out]
                n117 = Re/Im To Polar(2:w263, 3:w264) -> (0:→"phase (cm/s)":sgl[][], 1:→"Vel mag (cm/s)":sgl[][])
                n118 = call "ColorWheelDoppler.vi"("clip value low (cm/s)"=w292, "clip value high (cm/s)"=w294, "vector"=w278) -> ("image"=→"Direction Map":picture)  [unwired: 8 in]
              }
            }
          }
          event "RMS": Value Change {
            n119 = event-data() -> ()  [unwired: 1 in, 1 out]
            n120 = Index Array(array=w302, index=w301) -> (element=w303:T15)
            n121 = Unbundle(w303) -> (w297:csg[][][], "Values"=w300:T9)  [unwired: 19 out]
            n122 = Multiply(x=w298, y=w297) -> (x*y=w296:cdb[][][])
            n123 = local read "z grid"() -> (w304:cdb[][])
            n124 = call "RMSE_Rotation.vi"("Values"=w300, "mask"=w299, "rev/s"="rev/s", "Coord Grid"=w304, "V m/s"=w296) -> ()  [unwired: 7 in]
          }
          event "Velocity  vs time (cm/s)": Cursor Move; "Card Cycles": Value Change {
            n125 = event-data() -> ()  [unwired: 1 in, 1 out]
            n126 = property on="Velocity  vs time (cm/s)" class="WFGraph (strict)"("Active Cursor"=0 ("Cursor.Cursor Index"), "Active Cursor"=1 ("Cursor.Cursor Index")) -> ("XScale.Multiplier"=w320:dbl, "Cursor.Cursor X"=w307:dbl, "Cursor.Cursor X"=w311:dbl)  [unwired: 2 in, 2 out]
            n127 = Index Array(array=w323, index=w321) -> (element=w322:T15)
            n128 = Unbundle(w322) -> ("Number of Frames"=w310:u32)  [unwired: 20 out]
            n129 = Divide(x=w307, y=w320) -> (x/y=w319:dbl)
            n130 = Subtract(x=w307, y=w311) -> (x-y=w318:dbl)
            n131 = Decrement(x=w310) -> (x-1=w324:u32)
            n132 = Absolute Value(x=w318) -> (abs(x)=w317:dbl)
            n133 = expression code="1000/x*60"(w317) -> (w316:dbl)
            n134 = In Range and Coerce(upper limit=w324, x=w319, lower limit=0.0 ("x")) -> (coerced(x)=w326:dbl)  [unwired: 1 out]
            n135 = Multiply(x=w316, y="Card Cycles") -> (x*y=→"BPM":dbl)
            n136 = property on="Plane" class="DigNum (strict)"("Val(Sgnl)"=w326) -> ()  [unwired: 2 in, 2 out]
            n137 = property on="Average vorticity vs time rot/s" class="WFGraph (strict)"("Active Cursor"=u32 0, "Cursor.Cursor X"=w307) -> ()  [unwired: 2 in, 2 out]
            n138 = property on="Simple Motion Tracker" class="WFGraph (strict)"("Cursor.Cursor X"=w307) -> ()  [unwired: 2 in, 2 out]
            n139 = property on="VelT" class="WFGraph (strict)"("Cursor.Cursor X"=w307) -> ()  [unwired: 2 in, 2 out]
          }
          event "mean vort", "vort frame  average", "center zero", "AVG #", "step vort", "vort min val": Value Change {
            n140 = event-data() -> ()  [unwired: 1 in, 1 out]
            n141 = Index Array(array=w355, index=w352) -> (element=w354:T15)
            n142 = Unbundle(w354) -> (w333:csg[][][], "Values"=w353:T9)  [unwired: 19 out]
            n143 = Multiply(x=w331, y=w333) -> (x*y=w332:cdb[][][])
            n144 = property on="Vel Y (cm/s) Main" class="IntGraph (strict)"("Active Cursor"=1, "Active Cursor"=2) -> ("Cursor.Cursor Position"=w360:T8, "Cursor.Cursor Position"=w361:T8)  [unwired: 2 in, 2 out]
            n145 = property on="Velocity  vs time (cm/s)" class="WFGraph (strict)"() -> ("XScale.Multiplier"=w330:dbl)  [unwired: 2 in, 2 out]
            n146 = Bundle("center zero"="center zero", "center zero"="center zero") -> (w341:cluster{"center zero":i32, "center zero":i32})  [unwired: 1 in]
            n147 = local read "No Mask?"() -> (w340:bool)
            n148 = local read "y scale Circ"() -> (w349:sgl)
            n149 = Build Array(w360, w361, w341) -> (w350:T8[])
            n150 = call "AverageVorticity.vi"("AVG#"="AVG #", "step vort"="step vort", "v average"="vort frame  average", "Mean/Median"="Vort Mean/Median", "No Mask?"=w340, "Velocity field"=w332, "Values"=w353, "y scale"=w349, "vort min val"="vort min val", "Cursor positions"=w350) -> ("Energy loss v time in window"=→"Energy loss vs time in window":dbl[], "KE vs time"=→"KE vs time":dbl[], "Average vorticity v time rad/s"=w329:dbl[][], "All vorticity"=w357:dbl[][][])  [unwired: 2 in]
            "Average vorticity vs time rot/s" <- w329
            n151 = property on="Energy loss vs time in window" class="WFGraph (strict)"("XScale.Multiplier"=w330) -> ()  [unwired: 2 in, 2 out]
            n152 = property on="Average vorticity vs time rot/s" class="WFGraph (strict)"("XScale.Multiplier"=w330) -> ()  [unwired: 2 in, 2 out]
            n153 = Index Array(array=w329) -> (element=w328:dbl[])  [unwired: 2 in]
            n154 = call-poly <vilib>:"Mean.vi"("X"=w328) -> ("mean"=w348:dbl)  [unwired: 1 out]
            "mean vorticity" <- w348
            n155 = local read "rev/s"() -> (w346:dbl)
            n156 = Subtract(x=w348, y=w346) -> (x-y=w347:dbl)
            n157 = Divide(x=w347, y=w346) -> (x/y=w345:dbl)
            n158 = Multiply(x=w345, y=100.0) -> (x*y=→"error%":dbl)
          }
          event "Frame": Value Change {
            n159 = event-data() -> ("NewVal"=w373:i32)  [unwired: 1 in]
            n160 = Index Array(array=w376, index=w377) -> (element=w378:T15)
            n161 = Unbundle(w378) -> (w364:csg[][][])  [unwired: 20 out]
            n162 = property on="Vel Y (cm/s) Main" class="IntGraph (strict)"("Active Cursor"=2, "Active Cursor"=1) -> ("Cursor.Cursor Position"=w385:T8, "Cursor.Cursor Position"=w386:T8)  [unwired: 2 in, 2 out]
            n163 = Unbundle By Name(w386) -> ("Cursor X"=w381:dbl, "Cursor Y"=w382:dbl)
            n164 = Unbundle By Name(w385) -> ("Cursor X"=w383:dbl, "Cursor Y"=w384:dbl)
            n165 = Multiply(x=w363, y=w364) -> (x*y=w362:cdb[][][])
            n166 = Subtract(x=w382, y=w384) -> (x-y=w388:dbl)
            n167 = Subtract(x=w381, y=w383) -> (x-y=w387:dbl)
            n168 = Array Subset(array=w362, index (dim 1)=w383, length (dim 1)=w387, index (dim 2)=w384, length (dim 2)=w388) -> (w374:cdb[][][])  [unwired: 2 in]
            n169 = Index Array(array=w374, index (dim 0)=w373) -> (element=w371:cdb[][])  [unwired: 2 in]
            n170 = Array Size(array=w371) -> (size(s)=w372:i32[])
            n171 = Multiply Array Elements(1:w372) -> (0:w369:i32)
            n172 = Reshape Array(w371, w369) -> (w370:cdb[])
            n173 = Complex To Re/Im(x + iy=w370) -> (x=w368:dbl[], y=w366:dbl[])
            n174 = call "Convert to Dynamic Data"("Array"=w368) -> ("Dynamic Data Type"=w367:dynamicdata)  [unwired: 3 in]
            n175 = call "Convert to Dynamic Data2"("Array"=w366) -> ("Dynamic Data Type"=w365:dynamicdata)  [unwired: 3 in]
            n176 = call "Build XY Graph"("Y Input"=w365, "X Input"=w367) -> ("XY Graph"=→"Velocity spread":cluster{"X":dbl[], "Y":dbl[]}[])  [unwired: 8 in, 1 out]
          }
          event "Save Vortex": Value Change {
            n177 = event-data() -> ()  [unwired: 1 in, 6 out]
            n178 = Index Array(array=w431, index=w411) -> (element=w432:T15)
            n179 = Unbundle(w432) -> ("appended path"=w425:path, w401:sgl[][][])  [unwired: 19 out]
            n180 = property on="Average vorticity vs time rot/s" class="WFGraph (strict)"() -> ("XScale.Multiplier"=w435:dbl)  [unwired: 2 in, 2 out]
            n181 = Strip Path(path=w425) -> (stripped path=w424:path, name=w392:string)
            n182 = Array Size(array=w401) -> (size(s)=w400:i32[])
            n183 = Search and Replace String(input string=w392, search string="_B1") -> (result string=w404:string, offset past replacement=w398:i32)  [unwired: 6 in, 2 out]
            n184 = Index Array(array=w400) -> (element=w399:i32)  [unwired: 1 in]
            n185 = local read "Average vorticity vs time rot/s"() -> (w436:dbl[][])
            n186 = for {
              N: w399 -> [_]
              tunnel: w435 -> [w446]
              tunnel: [w445] -> w421 mode=indexing
              i -> [w447]
              n187 = Multiply(x=w446, y=w447) -> (x*y=w445:dbl)
            }
            n188 = Greater Than 0?(x=w398) -> (x > 0?=w397:bool)
            n189 = local read "Energy loss vs time in window"() -> (w437:dbl[])
            n190 = Search and Replace String(input string=w404, search string="raw", replace string="txt" ("replace string (\"\")")) -> (result string=w395:string)  [unwired: 5 in, 3 out]
            n191 = Search and Replace String(input string=w395, search string="CD") -> (result string=w394:string)  [unwired: 6 in, 3 out]
            n192 = local read "Simple Motion Tracker"() -> (w402:dbl[])
            n193 = local read "KE vs time"() -> (w418:dbl[])
            n194 = Select(t=500.0, s=w397, f=0.0) -> (s? t:f=w405:dbl)
            n195 = Add(x=w405, y=w421) -> (x+y=w409:dbl[])
            n196 = Concatenate Strings("vort add char", "VortMotion_" ("string"), w394) -> (w427:string)
            n197 = Build Array (concatenate)(w409, w436, w437, w418, w402) -> (w410:dbl[][])
            n198 = Build Path(base path=w424, name or relative path=w427) -> (appended path=w426:path)
            n199 = for {
              tunnel: w410 -> [w443] mode=indexing
              tunnel: [w444] -> w408 mode=indexing
              tunnel: "downsamp factor" -> [w442]
              n200 = call-poly <vilib>:"Decimate (single shot).vi"("decimating factor"=w442, "X"=w443) -> ("Decimated Array"=w444:dbl[])  [unwired: 8 in, 1 out]
            }
            n201 = property on="Vel Y (cm/s) Main" class="IntGraph (strict)"("Active Cursor"=u32 1, "Active Cursor"=u32 2) -> ("Cursor.Cursor Position"=w433:T8, "Cursor.Cursor Position"=w416:T8)  [unwired: 2 in, 2 out]
            n202 = Cluster To Array(cluster=w416) -> (array=w414:dbl[])
            n203 = Cluster To Array(cluster=w433) -> (array=w415:dbl[])
            n204 = Transpose 2D Array(2D array=w408) -> (transposed array=w423:dbl[][])
            n205 = Build Array (concatenate)(w415, w414) -> (w413:dbl[])
            n206 = case shown="False" w397 {
              tunnel: w423 -> [w440 w441]
              tunnel: [w439 w441] -> w422
              tunnel: w413 -> [w438 _]
              frame False {
                n207 = Build Array (concatenate)(w438, w440) -> (w439:dbl[][])
              }
              frame True {
              }
            }
            n208 = call-poly <vilib>:"Write Delimited Spreadsheet.vi"("file path (dialog if empty)"=w426, "format (%.3f)"="%.3e", "2D data"=w422, "append to file? (new file:F)"=w397) -> ()  [unwired: 10 in, 2 out]
          }
          event "SG Fix", "B1 Set", "VPI Fix", "CD Fix": Value Change {
            n209 = event-data() -> ()  [unwired: 1 in, 1 out]
            n210 = stacked-sequence {
              seq-local: [w495 _ _ _] -> [_ _ _ w646]
              tunnel: w453 -> [w519 w582 w615 _]
              tunnel: w452 -> [w516 w580 w614 _]
              tunnel: w451 -> [_ _ _ w649]
              tunnel: w450 -> [w497 _ w612 _]
              tunnel: [_ _ w612 _] -> w449
              tunnel: w448 -> [w456 w563 _ _]
              frame #0 {
                w481 = T11 0 items=["no dialog", "OK message", "continue or stop message", "OK message + warnings", "continue/stop + warnings"] ("type of dialog (OK msg:1)")
                w526 = 100
                n211 = Index Array(array=w519, index=w516) -> (element=w518:T15)
                n212 = Unbundle(w518) -> ("AVI Refnum (duplicate)"=w499:T13, "New Image"=w517:T5, "appended path"=w484:path, w458:csg[][][], "AVI Refnum (duplicate)"=w514:T13, "New Image"=w513:T5, "Number of Frames"=w503:u32, "Number of Frames"=w508:u32, "result string"=w483:string)  [unwired: 12 out]
                n213 = local read "Plane"() -> (w472:i32)
                n214 = Search and Replace String(input string=w483, search string="_B1") -> (offset past replacement=w491:i32)  [unwired: 6 in, 3 out]
                n215 = property on="Vel Y (cm/s) Main" class="IntGraph (strict)"("Active Cursor"=u32 0) -> ("Cursor.Cursor Position"=w495:T8)  [unwired: 2 in, 2 out]
                n216 = Decrement(x=w503) -> (x-1=w504:u32)
                n217 = Decrement(x=w508) -> (x-1=w509:u32)
                n218 = Greater Than 0?(x=w491) -> (x > 0?=w490:bool)
                n219 = In Range and Coerce(upper limit=w504, x=w472, lower limit=0) -> (coerced(x)=w505:u32)  [unwired: 1 out]
                n220 = In Range and Coerce(upper limit=w509, x=w472, lower limit=0) -> (coerced(x)=w507:u32)  [unwired: 1 out]
                n221 = Array Size(array=w497) -> (size(s)=w512:i32[])
                n222 = Strip Path(path=w484) -> (stripped path=w485:path)  [unwired: 1 out]
                n223 = Build Path(base path=w485, name or relative path=w483) -> (appended path=w482:path)
                n224 = call "Read_SG_JPG.vi"("Plane"=w472, "Scale cluster"="SG Fix", "B1 Set"=w490, "Array Dims"=w512, "in coordinates"=w495, "directory path"=w482) -> ("SG"=→"SG":picture, "concatenated string"=→"SG File":string)  [unwired: 4 in]
                n225 = call "IMAQ AVI2 Read Frame"("Frame Number"=w505, "Image"=w517, "AVI Refnum"=w499) -> ("error out"=w480:errorcluster, "Image Out"=w523:T5)  [unwired: 1 in, 6 out]
                n226 = call "OverlayCrossHatch.vi"("VPI"="VPI Fix", "error in (no error)"=w480, "Array Size"=w512, "Cursor Coord"=w495, "Vector Image"=w523) -> ("error out"=w479:errorcluster, "Point Location"=w522:cluster{dbl, dbl}[])  [unwired: 5 in]
                n227 = Unbundle By Name(w495) -> ("Cursor X"=w471:dbl, "Cursor Y"=w470:dbl)
                n228 = property on="Raw data (motion track marks)" class="IntGraph (strict)"("Active Cursor"=u32 0, "Cursor.Cursor Position"=w495) -> ()  [unwired: 2 in, 2 out]
                n229 = call "Overlay Feature Points.vi"("error in"=w479, "Feature Points"=w522, "Image"=w523) -> ("error out"=w478:errorcluster, "Image Out"=→"Vector Image":T5)  [unwired: 7 in]
                n230 = call "IMAQ AVI2 Read Frame"("error in (no error)"=w478, "Frame Number"=w507, "Image"=w513, "AVI Refnum"=w514) -> ("error out"=w477:errorcluster, "Image Out"=w515:T5)  [unwired: 6 out]
                n231 = call "OverlayCrossHatch.vi"("VPI"="CD Fix", "error in (no error)"=w477, "Array Size"=w512, "Cursor Coord"=w495, "Vector Image"=w515) -> ("error out"=w476:errorcluster, "Point Location"=w492:cluster{dbl, dbl}[])  [unwired: 5 in]
                n232 = property on="Vel X (cm/s) Ref" class="IntGraph (strict)"("Cursor.Cursor Position"=w495) -> ()  [unwired: 2 in, 2 out]
                n233 = Subtract(x="length", y=10) -> (x-y=w460:i32)
                n234 = local read "Operation"() -> (w474:u16)
                n235 = local read "AVG"() -> (w473:i32)
                n236 = Index Array(array=w458, index (dim 0)=w472, index (dim 2)=w470) -> (element=w488:csg[])  [unwired: 1 in]
                n237 = Index Array(array=w458, index (dim 0)=w472, index (dim 1)=w471) -> (element=w486:csg[])  [unwired: 1 in]
                n238 = call "Overlay Feature Points.vi"("error in"=w476, "Feature Points"=w492, "Image"=w515) -> ("error out"=w475:errorcluster, "Image Out"=→"CD Image":T5)  [unwired: 7 in]
                n239 = Array Subset(array=w458, index (dim 0)=w472, length (dim 0)=w460) -> (w457:csg[][][])  [unwired: 4 in]
                n240 = property on="Vel Y (cm/s) Ref" class="IntGraph (strict)"("Cursor.Cursor Position"=w495) -> ()  [unwired: 2 in, 2 out]
                n241 = Multiply(x=w456, y=w488) -> (x*y=w487:cdb[])
                n242 = Multiply(x=w456, y=w486) -> (x*y=w454:cdb[])
                n243 = Multiply(x=w456, y=w457) -> (x*y=w455:cdb[][][])
                n244 = for {
                  tunnel: w455 -> [w552] mode=indexing
                  tunnel: w474 -> [w551]
                  tunnel: w473 -> [w550]
                  tunnel: w471 -> [w547]
                  tunnel: w470 -> [w546]
                  tunnel: "length" -> [w545]
                  tunnel: [w541] -> w468 mode=indexing
                  n245 = Complex To Re/Im(x + iy=w552) -> (x=w554:dbl[][], y=w553:dbl[][])
                  n246 = call "MedianFilter2D.vi"("Operation"=w551, "Pts to use"=w550, "Raw In"=w553) -> ("output array"=w548:sgl[][])  [unwired: 8 in]
                  n247 = call "MedianFilter2D.vi"("Operation"=w551, "Pts to use"=w550, "Raw In"=w554) -> ("output array"=w549:sgl[][])  [unwired: 8 in]
                  n248 = Re/Im To Complex(1:w548, 2:w549) -> (0:w540:csg[][])
                  n249 = Array Subset(array=w540, index (row)=w547, length (row)=w545, index (col)=w546, length (col)=w545) -> (w538:csg[][])
                  n250 = Absolute Value(x=w538) -> (abs(x)=w539:sgl[][])
                  n251 = Array Max & Min(array=w539) -> (max index (indices)=w544:i32[])  [unwired: 3 out]
                  n252 = Index Array(array=w544) -> (element #1=w543:i32, element #2=w542:i32)  [unwired: 2 in]
                  n253 = Index Array(array=w538, index (row)=w543, index (col)=w542) -> (element=w541:csg)
                }
                n254 = Build Array(w454, w487) -> (w536:cdb[][])
                n255 = Index Array(array=w454, index=w470) -> (element=w528:cdb)
                n256 = Multiply(x=w528, y=w526) -> (x*y=w527:cdb)
                n257 = Multiply(x=w536, y=w526) -> (x*y=w537:cdb[][])
                n258 = call <vilib>:"Simple Error Handler.vi"("type of dialog (OK msg:1)"=w481, "error in (no error)"=w475) -> ()  [unwired: 3 in, 5 out]
                n259 = Complex To Polar(r * e^(i*theta)=w537) -> (r=→"Velocity cut x-y plane (cm/s)":dbl[][])  [unwired: 1 out]
                n260 = Complex To Polar(r * e^(i*theta)=w527) -> (r=w534:dbl, theta=w531:dbl)
                n261 = expression code="x*180/3.1419"(w531) -> (w530:dbl)
                n262 = Complex To Re/Im(x + iy=w527) -> (x=w533:dbl, y=w532:dbl)
                n263 = Absolute Value(x=w468) -> (abs(x)=w469:sgl[])
                n264 = Array Max & Min(array=w469) -> (max index (indices)=w467:i32)  [unwired: 3 out]
                n265 = Index Array(array=w468, index=w467) -> (element=w464:csg)
                n266 = Multiply(x=w464, y=100) -> (x*y=w462:csg)
                n267 = Complex To Polar(r * e^(i*theta)=w462) -> (r=w502:sgl, theta=w501:sgl)
                n268 = expression code="x*180/3.1419"(w501) -> (w500:sgl)
                n269 = Complex To Re/Im(x + iy=w462) -> (x=w466:sgl, y=w465:sgl)
                n270 = Bundle(w533, w532, w534, w530, w466, w465, w502, w500, "Cursor X"=w471, "Cursor Y"=w470, "Plane"=w472) -> (→"Vel Sum (cm/s)":T18)  [unwired: 1 in]
              }
              frame #1 {
                w561 = 15 ("index")
                w591 = 5
                n271 = property on="Vel Y (cm/s) Main" class="IntGraph (strict)"("Active Cursor"=u32 0) -> ("Cursor.Cursor Position"=w583:T8)  [unwired: 2 in, 2 out]
                n272 = Index Array(array=w582, index=w580) -> (element=w581:T15)
                n273 = Unbundle By Name(w583) -> ("Cursor X"=w556:dbl, "Cursor Y"=w567:dbl)
                n274 = Unbundle(w581) -> (w566:csg[][][], w568:sgl[][][])  [unwired: 19 out]
                n275 = Index Array(array=w568, index (dim 1)=w556, index (dim 2)=w567) -> (element=w562:sgl[])  [unwired: 1 in]
                n276 = Index Array(array=w566, index (dim 1)=w556, index (dim 2)=w567) -> (element=w565:csg[])  [unwired: 1 in]
                n277 = Initialize Array(0.0 ("element"), w561) -> (w559:dbl[])
                n278 = Array Subset(array=w562, index=w561) -> (w558:sgl[])  [unwired: 1 in]
                n279 = Multiply(x=w563, y=w565) -> (x*y=w564:cdb[])
                n280 = Build Array (concatenate)(w559, w558) -> (→"VelT":dbl[])
                n281 = property on="Velocity  vs time (cm/s)" class="WFGraph (strict)"() -> ("XScale.Multiplier"=w555:dbl)  [unwired: 2 in, 2 out]
                n282 = Multiply(x=w564, y=100) -> (x*y=w575:cdb[])
                n283 = expression code="2*x"(w591) -> (w593:i32)
                n284 = Array Size(array=w575) -> (size(s)=w594:i32)
                n285 = Subtract(x=w594, y=w593) -> (x-y=w592:i32)
                n286 = local read "AVG"() -> (w569:i32)
                n287 = Array Subset(array=w575, index=w591, length=w592) -> (w573:cdb[])
                n288 = property on="VelT" class="WFGraph (strict)"("XScale.Multiplier"=w555) -> ()  [unwired: 2 in, 2 out]
                n289 = for {
                  tunnel: w573 -> [_] mode=indexing
                  tunnel: w569 -> [w597]
                  tunnel: w573 -> [w600]
                  tunnel: [w596] -> w570 mode=indexing
                  i -> [w601]
                  n290 = Array Subset(array=w600, index=w601, length=w597) -> (w599:cdb[])
                  n291 = Add Array Elements(numeric array=w599) -> (sum=w598:cdb)
                  n292 = Divide(x=w598, y=w597) -> (x/y=w596:cdb)
                }
                n293 = Complex To Polar(r * e^(i*theta)=w573) -> (r=w590:dbl[], theta=w589:dbl[])
                n294 = Complex To Re/Im(x + iy=w573) -> (x=w595:dbl[], y=w579:dbl[])
                n295 = case shown="False" FALSE {
                  tunnel: w589 -> [_ w607]
                  tunnel: w579 -> [_ w606]
                  frame False {
                  }
                  frame True {
                    n296 = call "PhaseMapShift.vi"("V_y"=w606, "Phase"=w607) -> ()  [unwired: 8 in, 2 out]
                  }
                }
                n297 = Build Array(w590, w595, w579) -> (w572:dbl[][])
                n298 = Complex To Re/Im(x + iy=w570) -> (x=w586:dbl[], y=w585:dbl[])
                n299 = Complex To Polar(r * e^(i*theta)=w570) -> (r=w587:dbl[], theta=→"Flow Phase vs time":dbl[])
                n300 = Build Array(w587, w586, w585) -> (w577:dbl[][])
                "Velocity  vs time (cm/s)" <- w577
                n301 = for {
                  tunnel: w572 -> [w605] mode=indexing
                  tunnel: [w602] -> w571 mode=indexing
                  n302 = call <vilib>:"Std Deviation and Variance.vi"("X"=w605) -> ("mean"=w603:dbl, "variance"=w604:dbl)  [unwired: 1 in, 1 out]
                  n303 = Build Array(w603, w604) -> (w602:dbl[])
                }
                "V mean Var" <- w571
                n304 = for {
                  tunnel: w577 -> [w611] mode=indexing
                  tunnel: [w608] -> w576 mode=indexing
                  n305 = call <vilib>:"Std Deviation and Variance.vi"("X"=w611) -> ("mean"=w609:dbl, "variance"=w610:dbl)  [unwired: 1 in, 1 out]
                  n306 = Build Array(w609, w610) -> (w608:dbl[])
                }
                "V mean running" <- w576
              }
              frame #2 {
                n307 = case shown="False" FALSE {
                  tunnel: w615 -> [_ w620]
                  tunnel: w614 -> [_ w617]
                  frame False {
                  }
                  frame True {
                    n308 = Index Array(array=w620, index=w617) -> (element=w619:T15)
                    n309 = Unbundle(w619) -> (w618:csg[][][])  [unwired: 20 out]
                    n310 = property on="Vel Y (cm/s) Main" class="IntGraph (strict)"("Active Cursor"=u32 0) -> ("Cursor.Cursor Position"=w621:T8)  [unwired: 2 in, 2 out]
                    n311 = Unbundle By Name(w621) -> ("Cursor X"=w624:dbl, "Cursor Y"=w623:dbl)
                    n312 = Array Size(array=w618) -> (size(s)=w632:i32[])
                    n313 = Index Array(array=w632, index=2) -> (element=w629:i32)
                    n314 = Index Array(array=w632, index=1) -> (element=w628:i32)
                    n315 = for {
                      N: w628 -> [_]
                      tunnel: [w644] -> w627 mode=indexing
                      tunnel: w618 -> [w643]
                      tunnel: w624 -> [w640]
                      i -> [w642]
                      n316 = Index Array(array=w643, index (dim 1)=w640, index (dim 2)=w642) -> (element=w641:csg[])  [unwired: 1 in]
                      n317 = Absolute Value(x=w641) -> (abs(x)=w639:sgl[])
                      n318 = call-poly <vilib>:"Mean.vi"("X"=w639) -> ("mean"=w644:dbl)  [unwired: 1 out]
                    }
                    n319 = for {
                      N: w629 -> [_]
                      tunnel: [w638] -> w626 mode=indexing
                      tunnel: w618 -> [w637]
                      tunnel: w623 -> [w635]
                      i -> [w636]
                      n320 = Index Array(array=w637, index (dim 1)=w636, index (dim 2)=w635) -> (element=w634:csg[])  [unwired: 1 in]
                      n321 = Absolute Value(x=w634) -> (abs(x)=w633:sgl[])
                      n322 = call-poly <vilib>:"Mean.vi"("X"=w633) -> ("mean"=w638:dbl)  [unwired: 1 out]
                    }
                    n323 = Build Array(w627, w626) -> (w625:dbl[][])
                    n324 = expression code="x*100"(w625) -> (→"Velocity cut  mean\nall time(cm/s)":dbl[][])
                  }
                }
              }
              frame #3 {
                n325 = property on="Vel Y (cm/s) Main" class="IntGraph (strict)"("Active Cursor"=u32 1) -> ("Cursor.Cursor Position"=w645:T8)  [unwired: 2 in, 2 out]
                n326 = Subtract(x=w645, y=w646) -> (x-y=w647:T8)
                n327 = Unbundle By Name(w647) -> ("Cursor X"=w651:dbl, "Cursor Y"=w650:dbl)
                n328 = Index Array(array=w649, index (dim 1)=w651, index (dim 2)=w650) -> (element=w653:dbl[])  [unwired: 1 in]
                "Vorticity slow time" <- w653
                n329 = call-poly <vilib>:"Mean.vi"("X"=w653) -> ("mean"=→"vorticy pixel\nmean across time":dbl)  [unwired: 1 out]
              }
            }
          }
          event "True Center Freq": Value Change {
            n330 = event-data() -> ()  [unwired: 1 in, 4 out]
          }
          event "Raw data (motion track marks)": Cursor Move; "#x lines", "#y rf", "Ref Frame 2D CC": Value Change {
            n331 = event-data() -> ()  [unwired: 1 in, 4 out]
            n332 = Index Array(array=w675, index=w674) -> (element=w672:T15)
            n333 = Unbundle(w672) -> (w665:sgl[][][])  [unwired: 20 out]
            n334 = property on="Raw data (motion track marks)" class="IntGraph (strict)"("Active Cursor"=u32 1) -> ("Cursor.Cursor Position"=w669:T8)  [unwired: 2 in, 2 out]
            n335 = call "MotionTracker2DCorr.vi"("Ref frame for 2S"="Ref Frame 2D CC", "Cursor.Cursor Position"=w669, "#x lines"="#x lines", "#y rf"="#y rf", "RF In"=w665, "2D threshold"="2D threshold") -> ("Mean axial Disp"=w657:dbl[], "2D corr"=→"2D Correlation":dbl[][], "Peak tracker"=→"Peak Tracker":dbl[][])  [unwired: 3 in]
            "Simple Motion Tracker" <- w657
            n336 = Build Array(w657) -> (w661:dbl[][])
            n337 = call "SubMean.vi"("Bit Depth"=50, "Scan Data In"=w661, "Type of Mean"=TypeofMean."Poly Mean") -> ("Array"=w660:dbl[][])  [unwired: 3 in, 2 out]
            n338 = Index Array(array=w660) -> ()  [unwired: 2 in, 1 out]
          }
          event "Save VPI JPGs": Value Change {
            n339 = event-data() -> ()  [unwired: 1 in, 4 out]
            n340 = Index Array(array=w696, index=w698) -> (element=w697:T15)
            n341 = Unbundle(w697) -> ("appended path"=w695:path)  [unwired: 20 out]
            n342 = Strip Path(path=w695) -> (stripped path=w691:path, name=w680:string)
            n343 = local read "Plane"() -> (w682:i32)
            n344 = Search and Replace String(input string=w680, search string="VPI_") -> (result string=w679:string)  [unwired: 6 in, 3 out]
            n345 = Search and Replace String(input string=w679, search string=".raw") -> (result string=w677:string)  [unwired: 6 in, 3 out]
            n346 = Number To Decimal String(number=w682) -> (decimal integer string=w693:string)  [unwired: 1 in]
            n347 = Concatenate Strings(w677, "_" ("string"), w693, ".jpg" ("replace string (\"\")")) -> (w685:string)
            n348 = Concatenate Strings("VPI_" ("replace string (\"\")"), w685) -> (w692:string)
            n349 = Concatenate Strings("CD_" ("replace string (\"\")"), w685) -> (w684:string)
            n350 = Build Path(base path=w691, name or relative path=w684) -> (appended path=w689:path)
            n351 = Build Path(base path=w691, name or relative path=w692) -> (appended path=w690:path)
            n352 = local read "Vector Image"() -> (w699:T5)
            n353 = local read "CD Image"() -> (w688:T5)
            n354 = call-poly "IMAQ Write File 2"("File Path"=w690, "Image"=w699) -> ()  [unwired: 8 in, 2 out]
            n355 = call-poly "IMAQ Write File 2"("File Path"=w689, "Image"=w688) -> ()  [unwired: 8 in, 2 out]
          }
          event "Save Vels": Value Change {
            w718 = "name\nnote\ntime (ms)\nx (pt)\ny (pt)\nmag (pt)\nphase (pt)\nx (mean)\ny (mean)\nmag (mean)\nphase (mean)\nCurs X\nCurs Y\nPlane (#)\nAVG (mean)"
            n356 = event-data() -> ()  [unwired: 1 in, 2 out]
            n357 = Index Array(array=w734, index=w733) -> (element=w732:T15)
            n358 = Unbundle(w732) -> ("appended path"=w731:path)  [unwired: 20 out]
            n359 = property on="Velocity  vs time (cm/s)" class="WFGraph (strict)"("Active Cursor"=0 ("Cursor.Cursor Index")) -> ("Cursor.Cursor X"=w710:dbl)  [unwired: 2 in, 2 out]
            n360 = local read "Vel Sum (cm/s)"() -> (w726:T7)
            n361 = Strip Path(path=w731) -> (name=w702:string)  [unwired: 1 out]
            n362 = Search and Replace String(input string=w702, search string="_B1") -> (offset past replacement=w703:i32)  [unwired: 6 in, 3 out]
            n363 = Greater Than 0?(x=w703) -> (x > 0?=w701:bool)
            n364 = Select(t=500.0, s=w701, f=0.0) -> (s? t:f=w705:dbl)
            n365 = Add(x=w710, y=w705) -> (x+y=w709:dbl)
            n366 = local read "AVG"() -> (w715:i32)
            n367 = Cluster To Array(cluster=w726) -> (array=w730:sgl[])
            n368 = Number To Fractional String(number=w709, precision (6)=i16 2) -> (F-format string=w711:string)  [unwired: 2 in]
            n369 = Number To Fractional String(number=w730, precision (6)=i16 2) -> (F-format string=w729:string[])  [unwired: 2 in]
            n370 = Number To Fractional String(number=w715, precision (6)=i16 2) -> (F-format string=w714:string)  [unwired: 2 in]
            n371 = Build Array (concatenate)(w702, "Location note", w711, w729, w714) -> (w722:string[])
            n372 = Spreadsheet String To Array(format string="%s", spreadsheet string=w718, array type (2D Dbl)=w718) -> (array=w719:string[][])  [unwired: 1 in]
            n373 = Index Array(array=w719, index (col)=0 ("disabled index (col)")) -> (element=w717:string[])  [unwired: 1 in]
            n374 = call <vilib>:"Check if File or Folder Exists.vi"("path"=path "D:/VPI.txt" ("file path (dialog if empty)")) -> ("file or folder exists?"=w723:bool, "dup path"=w724:path)  [unwired: 8 in, 1 out]
            n375 = stacked-sequence {
              tunnel: w724 -> [w737 w744]
              tunnel: w723 -> [w738 _]
              tunnel: w722 -> [_ w743]
              tunnel: w717 -> [w736 _]
              frame #0 {
                n376 = case shown="False" w738 {
                  tunnel: w737 -> [w740 _]
                  tunnel: w736 -> [w739 _]
                  frame False {
                    n377 = call-poly <vilib>:"Write Delimited Spreadsheet.vi"("file path (dialog if empty)"=w740, "1D data"=w739, "append to file? (new file:F)"=TRUE, "transpose? (no:F)"=FALSE) -> ()  [unwired: 10 in, 2 out]
                  }
                  frame True {
                  }
                }
              }
              frame #1 {
                n378 = call-poly <vilib>:"Write Delimited Spreadsheet.vi"("file path (dialog if empty)"=w744, "1D data"=w743, "append to file? (new file:F)"=TRUE, "transpose? (no:F)"=FALSE) -> ()  [unwired: 10 in, 2 out]
              }
            }
          }
          event "Short lag variance VarS": Cursor Move {
            n379 = event-data() -> ()  [unwired: 1 in, 1 out]
            n380 = Index Array(array=w752, index=w748) -> (element=w751:T15)
            n381 = Unbundle(w751) -> (w750:sgl[][][], w749:sgl[][][])  [unwired: 19 out]
            n382 = property on="Short lag variance VarS" class="IntGraph (strict)"() -> ("Cursor.Cursor X"=w757:dbl, "Cursor.Cursor Y"=w756:dbl)  [unwired: 2 in, 2 out]
            n383 = Index Array(array=w750, index (dim 1)=w757, index (dim 2)=w756) -> (element=→"powerFlow line":sgl[])  [unwired: 1 in]
            n384 = Index Array(array=w749, index (dim 1)=w757, index (dim 2)=w756) -> (element=→"Short lag vs slow time VarS":sgl[])  [unwired: 1 in]
          }
          event "VPI Case": Value Change {
            n385 = event-data() -> ("NewVal"=w786:i32)  [unwired: 1 in]
            n386 = Array Size(array=w785) -> (size(s)=w784:i32)
            n387 = local read "#x lines"() -> (w767:i32)
            n388 = local read "Plane"() -> (w791:i32)
            n389 = Decrement(x=w784) -> (x-1=w783:i32)
            n390 = In Range and Coerce(upper limit=w783, x=w786, lower limit=0) -> (coerced(x)=w782:i32)  [unwired: 1 out]
            n391 = property on="Plane" class="DigNum (strict)"("Val(Sgnl)"=w791) -> ()  [unwired: 2 in, 2 out]
            n392 = property on="#x lines" class="DigNum (strict)"("Val(Sgnl)"=w767) -> ()  [unwired: 2 in, 2 out]
            n393 = Index Array(array=w785, index=w782) -> (element=w793:T15)
            n394 = Unbundle(w793) -> ("appended path"=w792:path, "Values"=w775:T9, "mean pow"=→"Mean Pow":sgl[][], "mean var"=→"Mean varS":sgl[][], w766:sgl[][][], w765:sgl[][][])  [unwired: 15 out]
            n395 = Unbundle By Name(w775) -> ("skip"=w772:dbl)
            "Skip File" <- w772
            n396 = call "MeansOfData.vi"("var"=w765, "pow"=w766) -> ("mean pow"=w760:sgl[][])  [unwired: 7 in, 2 out]
            "Mean PowT" <- w760
            n397 = call-poly <vilib>:"Normalize.vi"("Matrix"=w760) -> ("Normalized Matrix"=w763:T19)  [unwired: 1 in, 3 out]
            n398 = Array Size(array=w760) -> (size(s)=w759:i32[])
            n399 = Strip Path(path=w792) -> (name=w777:string)  [unwired: 1 out]
            "Current  VPI" <- w777
            n400 = Multiply Array Elements(1:w759) -> (0:w758:i32)
            n401 = Reshape Array(w763, w758) -> (w762:dbl[])
            n402 = Match Pattern(string=w777, regular expression="D_") -> (after substring=w779:string)  [unwired: 1 in, 3 out]
            n403 = Select(t="Skip", s="Skip overide?", f=w772) -> (s? t:f=w771:dbl)
            n404 = Match Pattern(string=w779, regular expression="Hz") -> (before substring=w778:string)  [unwired: 1 in, 3 out]
            n405 = Decimal String To Number(string=w778) -> (number=w776:i32)  [unwired: 2 in, 1 out]
            n406 = call <vilib>:"Histogram.vi"("intervals"=20, "X"=w762) -> ("Histogram Graph"=→"Histogram Graph":T4)  [unwired: 6 in, 3 out]
            n407 = Divide(x=w776, y=w771) -> (x/y=w774:dbl)
            n408 = expression code="1000/x"(w774) -> (w773:dbl)
            n409 = property on="Velocity  vs time (cm/s)" class="WFGraph (strict)"("XScale.Multiplier"=w773) -> ()  [unwired: 2 in, 2 out]
          }
          event "EKG Trace": Value Change {
            n410 = event-data() -> ("NewVal"=w795:path)  [unwired: 1 in]
            n411 = call <vilib>:"Read BMP File.vi"("path to BMP file"=w795) -> ("image data"=w796:T20)  [unwired: 8 in, 2 out]
            n412 = call <vilib>:"Draw Flattened Pixmap.vi"("image data"=w796) -> ("new picture"=→"EKG":picture)  [unwired: 8 in]
          }
          event "Save Images": Value Change {
            w833 = TRUE ("Save?")
            n413 = event-data() -> ()  [unwired: 1 in, 1 out]
            n414 = Index Array(array=w848) -> (element=w847:T15)  [unwired: 1 in]
            n415 = Unbundle(w847) -> ("Header In"=w827:T1, "result string"=w800:string)  [unwired: 19 out]
            n416 = local read "Vel X (cm/s) Ref"() -> (w830:sgl[][])
            n417 = local read "Values"() -> (w843:T9)
            n418 = Search and Replace String(input string=w800, search string="_B1") -> (offset past replacement=w802:i32)  [unwired: 6 in, 3 out]
            n419 = Greater Than 0?(x=w802) -> (x > 0?=w801:bool)
            n420 = Unbundle By Name(w843) -> ("ystart"=w842:dbl, "deltaX"=w838:dbl, "deltaY"=w841:dbl)
            n421 = Array Size(array=w830) -> (size(s)=w846:i32[])
            n422 = Select(t=u32 500 ("Active Cursor"), s=w801, f=u32 0 ("Active Cursor")) -> (s? t:f=w805:u32)
            n423 = expression code="x*1000"(w841) -> (w835:dbl)
            n424 = property on="Velocity  vs time (cm/s)" class="WFGraph (strict)"("Active Cursor"=u32 0) -> ("Cursor.Cursor X"=w812:dbl)  [unwired: 2 in, 2 out]
            n425 = expression code="x*1000"(w842) -> (w839:dbl)
            n426 = expression code="x*1000"(w838) -> (w837:dbl)
            n427 = Index Array(array=w846, index #1=1 ("index"), index #2=0 ("index")) -> (element #1=w845:i32, element #2=w844:i32)
            n428 = Round To Nearest(number=w812) -> (nearest integer value=w806:dbl)
            n429 = Divide(x=750.0 ("y"), y=w835) -> (x/y=w840:dbl)
            n430 = Add(x=w806, y=w805) -> (x+y=w804:dbl)
            n431 = Number To Decimal String(number=w804) -> (decimal integer string=w811:string)  [unwired: 1 in]
            n432 = Bundle By Name(cluster=w827, "A/D info.# rf points per line"=w845, "A/D info.# lines per scan"=w844, "A/D info.sample rate MHz"=w840, "Scan Info.delay"=w839, "Scan Settings.Distance between\nscan lines (um)"=w837, "Misc Info.c speed"=i16 1500) -> (w826:T1)
            n433 = Concatenate Strings(w811, "Vector.jpg") -> (w819:string)
            n434 = Concatenate Strings(w811, "ColorDoppler.jpg") -> (w820:string)
            n435 = local read "CD Image"() -> (w831:T5)
            n436 = Concatenate Strings(w811, "xVel.eye") -> (w813:string)
            n437 = local read "Vector Image"() -> (w832:T5)
            n438 = Build Path(base path="ImageSavePath", name or relative path=w819) -> (appended path=w818:path)
            n439 = Build Path(base path="ImageSavePath", name or relative path=w820) -> (appended path=w822:path)
            n440 = Concatenate Strings(w811, "yVec.eye") -> (w815:string)
            n441 = local read "Vel Y (cm/s) Ref"() -> (w825:sgl[][])
            n442 = Build Path(base path="ImageSavePath", name or relative path=w813) -> (appended path=w824:path)
            n443 = Build Path(base path="ImageSavePath", name or relative path=w815) -> (appended path=w814:path)
            n444 = call-poly "IMAQ Write File 2"("File Path"=w818, "Image"=w832) -> ()  [unwired: 8 in, 2 out]
            n445 = call-poly "IMAQ Write File 2"("File Path"=w822, "Image"=w831) -> ()  [unwired: 8 in, 2 out]
            n446 = call "SaveDataSGLFast.vi"("Header In"=w826, "Save?"=w833, "Data Array"=w825, "File Name and Path"=w814) -> ()  [unwired: 7 in, 1 out]
            n447 = call "SaveDataSGLFast.vi"("Header In"=w826, "Save?"=w833, "Data Array"=w830, "File Name and Path"=w824) -> ()  [unwired: 7 in, 1 out]
          }
          event "Max V": Value Change {
            n448 = event-data() -> ("NewVal"=w854:i32)  [unwired: 1 in]
            n449 = Negate(x=w854) -> (-x=w853:i32)
            n450 = property on="Vel X (cm/s) Ref" class="IntGraph (strict)"("ZScale.Maximum"=w854, "ZScale.Minimum"=w853) -> ()  [unwired: 2 in, 2 out]
            n451 = property on="Vel Y (cm/s) Ref" class="IntGraph (strict)"("ZScale.Maximum"=w854, "ZScale.Minimum"=w853) -> ()  [unwired: 2 in, 2 out]
            n452 = property on="Vel mag (cm/s)" class="IntGraph (strict)"("ZScale.Maximum"=w854, "ZScale.Minimum"=0.0 ("Z Scale.Range:Minimum")) -> ()  [unwired: 2 in, 2 out]
            n453 = property on="Vel Y (cm/s) Main" class="IntGraph (strict)"("ZScale.Maximum"=w854, "ZScale.Minimum"=w853) -> ()  [unwired: 2 in, 2 out]
          }
        }
      }
    }
  }
  n454 = for {
    tunnel: w14 -> [w863] mode=indexing
    n455 = Unbundle(w863) -> ("AVI Refnum (duplicate)"=w862:T13, "New Image"=w861:T5, "AVI Refnum (duplicate)"=w859:T13, "New Image"=w858:T5)  [unwired: 17 out]
    n456 = call "IMAQ AVI2 Close"("AVI Refnum"=w859) -> ("error out"=w860:errorcluster)  [unwired: 1 in, 9 out]
    n457 = call "IMAQ AVI2 Close"("AVI Refnum"=w862) -> ("error out"=w864:errorcluster)  [unwired: 1 in, 9 out]
    n458 = call "IMAQ Dispose"("Image"=w858, "error in (no error)"=w860) -> ()  [unwired: 1 in, 4 out]
    n459 = call "IMAQ Dispose"("Image"=w861, "error in (no error)"=w864) -> ()  [unwired: 1 in, 4 out]
  }
